vi "Maize traits Extraction_English version.vi"() -> ()   [LabVIEW 2015]
uses:
  <vilib>/vision/Image Controls.llb/IMAQ Image.ctl
  <vilib>/Utility/file.llb/Read Delimited Spreadsheet (string).vi
  <vilib>/Utility/file.llb/Read From Spreadsheet File (string).vi
  <vilib>/Utility/file.llb/Write To Spreadsheet File (string).vi
  <vilib>/vision/NI_Vision_Development_Module.lvlib
  Realse/HistProperty.dll
  GLCM.dll
  <vilib>/Analysis/NI_AALBase.lvlib
  FTKToolkit_CPP_VC8.dll
  Realse/imFillRemove.dll
  TotalContoursConvexHull (5).dll
panel:
  out "Path of segmented images storage":path
  in  "Path of data sotrage":path=path "E:/文章投稿/51. 代明球老师-玉米胁迫实验/RGB程序/TEST"
  out "Barcode":string
  out "Path of input image":path=path "K:/玉米考种机上位机程序/12-255/13SD010-4.png"
  in  "Path of original images":path=path "E:/文章投稿/51. 代明球老师-玉米胁迫实验/RGB程序/TEST/Date.txt"
  out "Date":string
  out "LC上半部分均值":dbl format="%0.2f"
  out "LC上半部分标准差":dbl format="%0.2f"
  out "LC下半部分均值":dbl format="%0.2f"
  out "LC下半部分标准差":dbl format="%0.2f"
  out "叶尖点到结点长度上半部分均值":dbl format="%0.2f"
  out "叶尖点到结点长度上半部分标准差":dbl format="%0.2f"
  out "叶尖点到结点长度下半部分均值":dbl format="%0.2f"
  out "叶尖点到结点长度下半部分标准差":dbl format="%0.2f"
  out "LC均值":dbl format="%0.2f"
  out "LC标准差":dbl format="%0.2f"
  out "叶尖点到结点总长":dbl
  out "叶尖点到结点长度均值":dbl format="%0.2f"
  out "叶尖点到结点长度标准差":dbl format="%0.2f"
  out "steamWidth":dbl
  out "leafEndToEndDistance":dbl[](array[numeric])
  out "unsigned 8bit integer":u8
  out "deleted portion":dbl[](array[numeric])
  out "array w/ subset deleted":dbl[](array[numeric])
  out "拉直后叶长上半部分均值":dbl format="%0.2f"
  out "拉直后叶长上半部分标准差":dbl format="%0.2f"
  out "拉直后叶长下半部分均值":dbl format="%0.2f"
  out "拉直后叶长下半部分标准差":dbl format="%0.2f"
  out "叶片角度2上半部分均值":dbl format="%0.2f"
  out "叶片角度2上半部分标准差":dbl format="%0.2f"
  out "叶片角度2下半部分均值":dbl format="%0.2f"
  out "叶片角度2下半部分标准差":dbl format="%0.2f"
  out "叶片角度1下半部分均值":dbl format="%0.2f"
  out "叶片角度1下半部分标准差":dbl format="%0.2f"
  out "叶片角度1上半部分均值":dbl format="%0.2f"
  out "叶片角度1上半部分标准差":dbl format="%0.2f"
  out "拉直后叶长标准差":dbl format="%0.2f"
  out "拉直后叶长均值":dbl format="%0.2f"
  out "拉直后叶长总长":dbl
  out "叶片角度2总长":dbl format="%0.2f"
  out "叶片角度2标准差":dbl format="%0.2f"
  out "叶片角度1总长(切线)":dbl format="%0.2f"
  out "叶片角度1标准差(切线)":dbl format="%0.2f"
  out "结点长标准差":dbl format="%0.2f"
  out "结点长均值":dbl format="%0.2f"
  out "结点总长":dbl
  out "Convex Hull image":T1(plugin-control)
  out "Gradient image of green component":T1(plugin-control)
  out "leafLength":dbl[](array[numeric])
  out "nodePointPosition":u32[](array[numeric])
  out "leafAngle2":dbl[](array[numeric])
  out "leafAngle1":dbl[](array[numeric])
  out "inputLeafEndPoint":u32[](array[numeric])
  out "outputLeafNum":u32
  out "Area/convex hull area":dbl
  out "Type":dbl
  out "Heywood":dbl
  out "Compactness":dbl
  out "Elongation":dbl
  out "Type_convex hull":dbl
  out "Heywood_convex hull":dbl
  out "Compactness_convex hull":dbl
  out "Elongation_convex hull":dbl
  out "Perimeter_convex hull":dbl
  out "Area_convex hull":dbl
  out "T":sgl[](array[numeric])=[0.2502537, 0.67057997, 5.4486604, 0.09361785, 0.21617743, 888061250.0, 3.9959273, 60957.523, 1.6065311, -402198.06, 2.7884297, 7.334512, 0.26611477, 1.6175103, 60956.69]
  in  "level":i32=16
  out "HistStat_I":dbl[](array[numeric])
  out "HistStat_S":dbl[](array[numeric])
  out "HistStat_G":dbl[](array[numeric])
  out "HistStat_H":dbl[](array[numeric])
  out "GCV2":dbl
  out "HWR":dbl
  out "PP":dbl
  out "FDIC":sgl
  out "TPA":dbl
  out "TBR":dbl
  out "FDNIC":sgl
  out "MPH":dbl
  out "PW":dbl
  out "PAR":dbl
  out "PC1-PC6":sgl[](array[numeric])
  in  "Range":cluster{"Lower value":sgl, "Upper value":sgl}={"Lower value"=110.0, "Upper value"=255.0}
  out "filenames":string[](array[string])
  out "max index(es)":i32
  in  "Removeareathreshold":i32=1000
  in  "EGthreshold":sgl=0.15
  in  "ERthreshold":sgl=0.5
  out "20 side-view images":T1(plugin-control)
  out "Numeric":i32
  out "Original image with maximum plant width":T1(plugin-control)
  out "Segmented image":T1(plugin-control)
  # "Maize Phenotypic traits Extraction"
  # "Plant Traits"
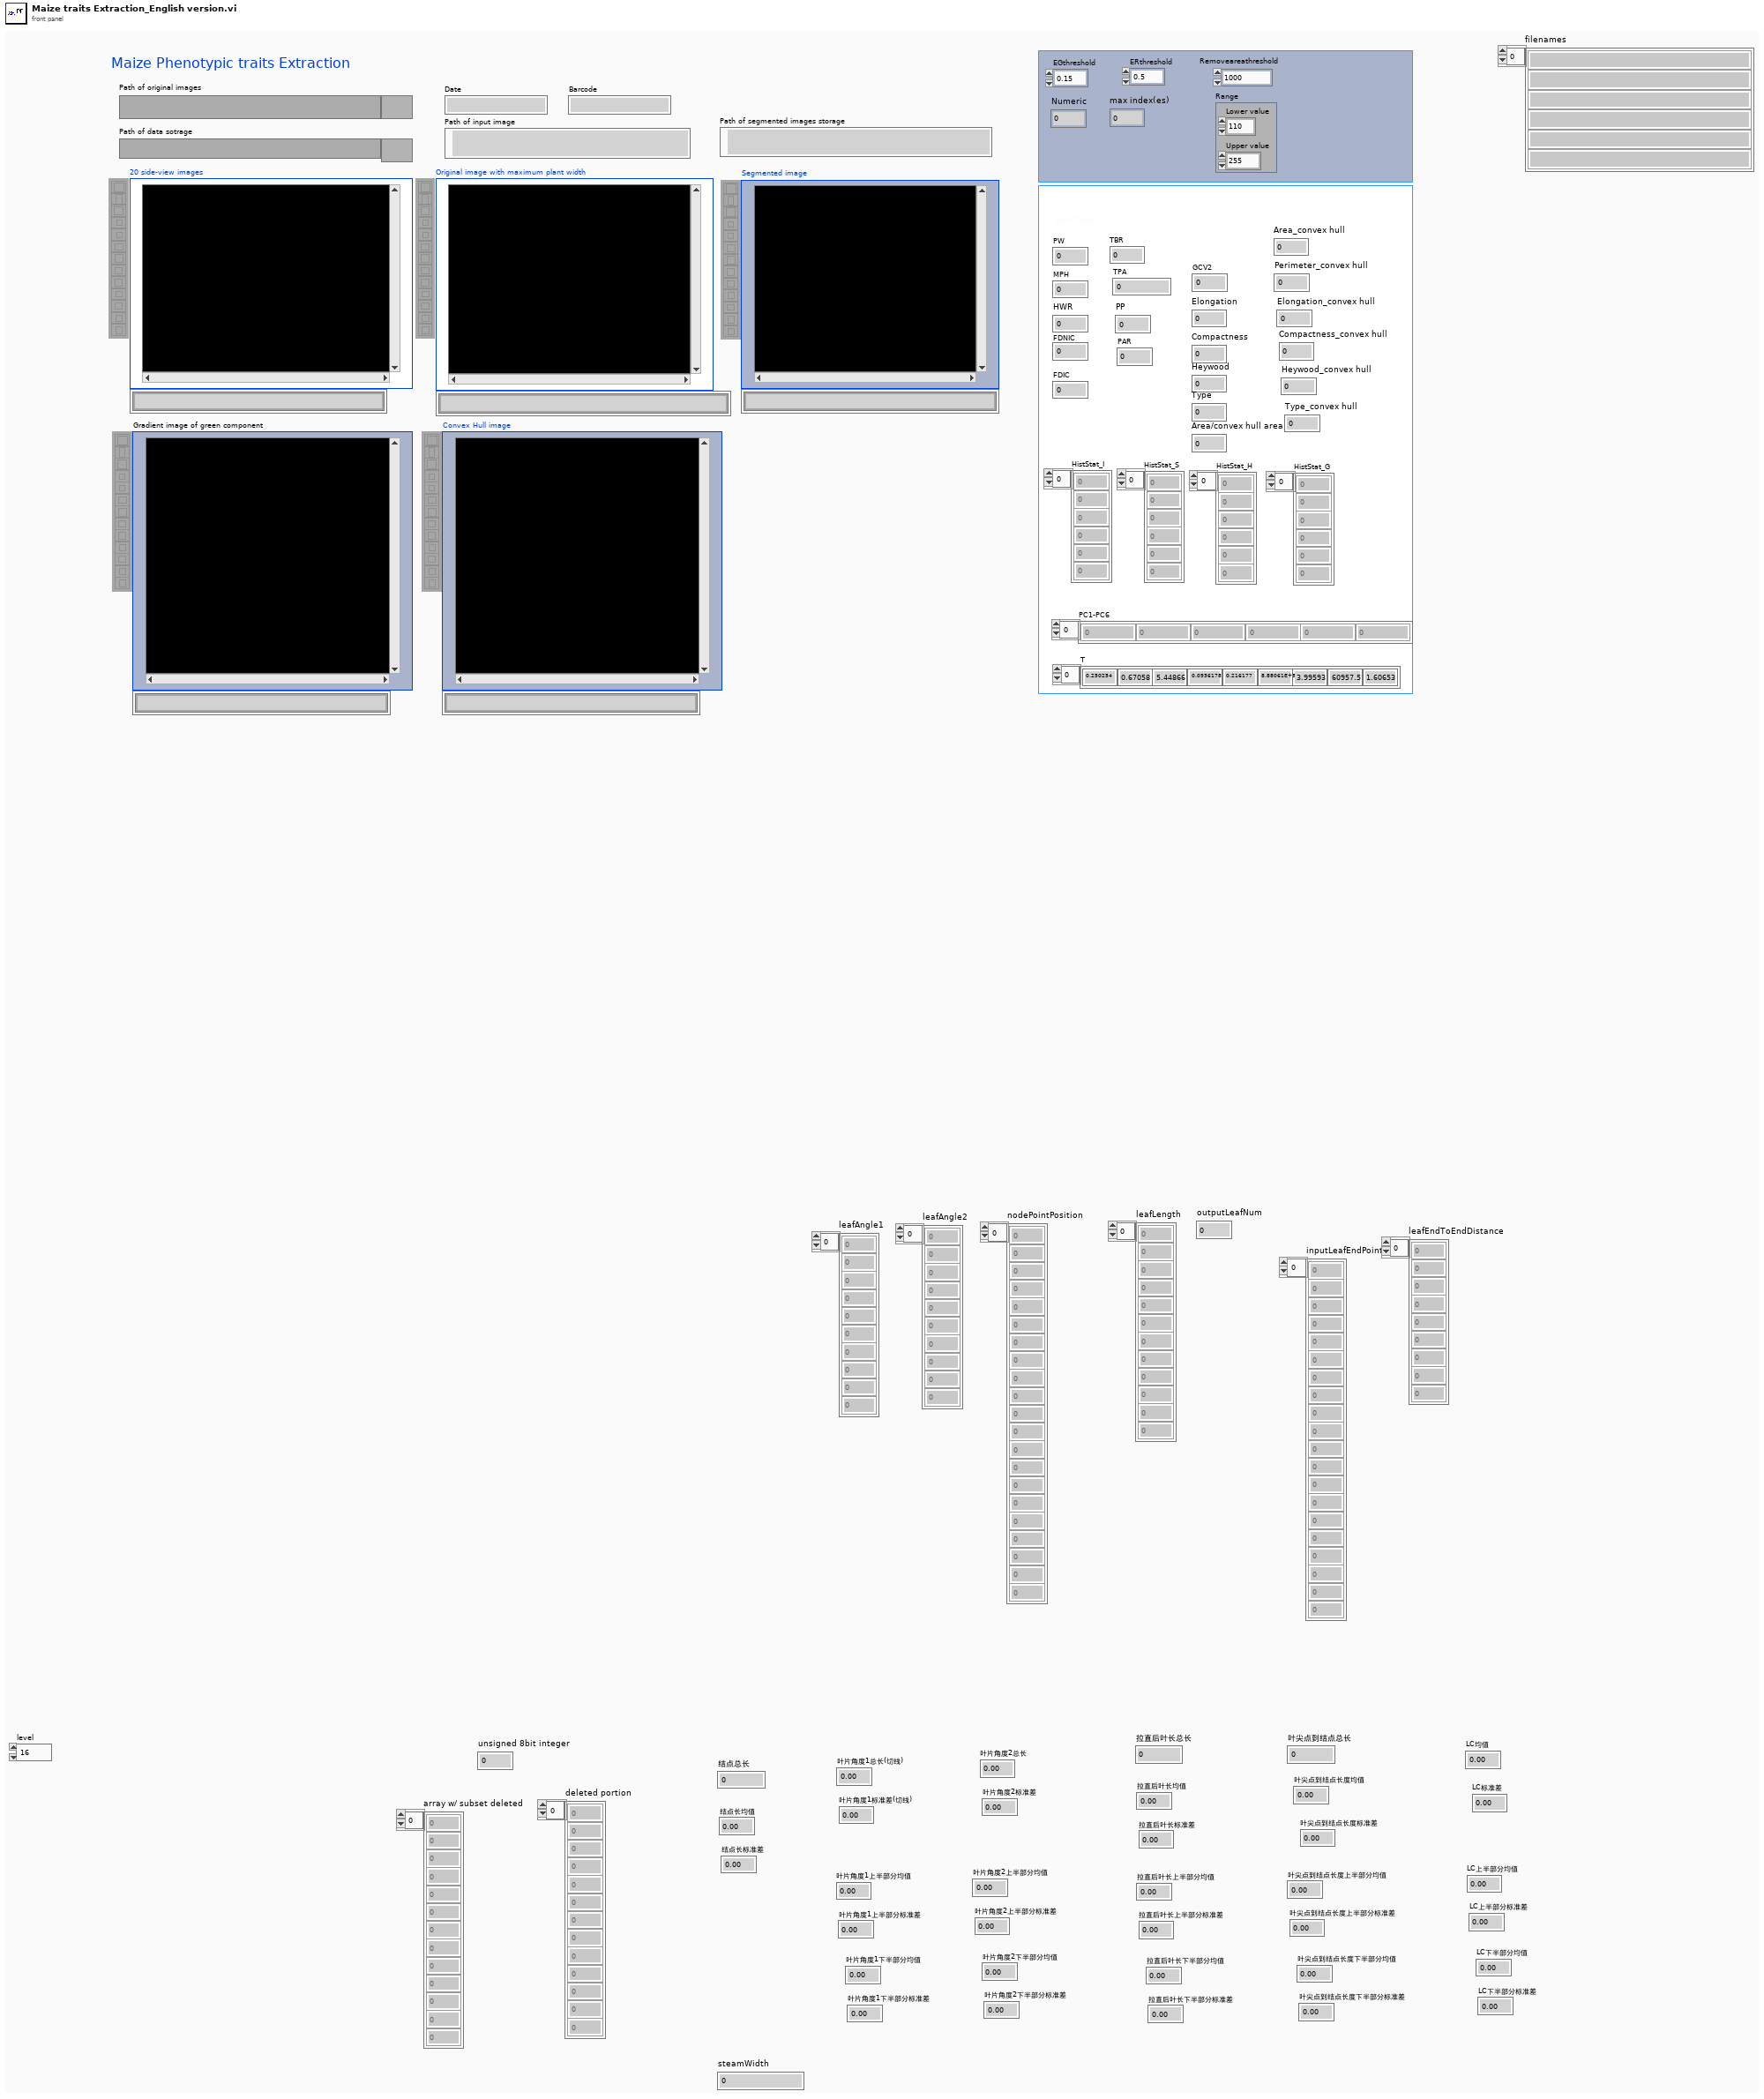
[diagram p1: front panel]
types:
  T1 = typedef "IMAQ Image.ctl" = refnum<image>
  T2 = enum32{"AutoM", "Close", "Dilate", "Erode", "Gradient", "Gradient out", "Gradient in", "Hit miss", "Open", "PClose", "POpen", "Thick", "Thin"}
  T3 = enum32{"AutoM", "Close", "Dilate", "Erode", "Gradient", "Gradient in", "Gradient out", "HitMiss", "Open", "PClose", "POpen", "Thick", "Thin"}
  T4 = typedef "Image Type" = u32
  T5 = typedef "Particle Parameters" = i32
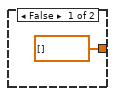
[diagram p2: hidden frame]
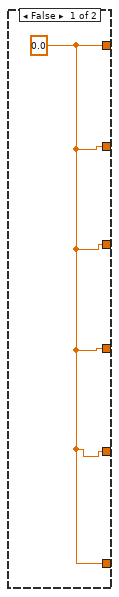
[diagram p3: hidden frame]
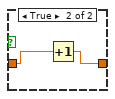
[diagram p7: hidden frame]
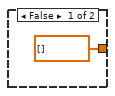
[diagram p8: hidden frame]
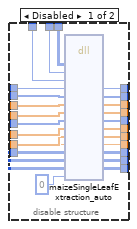
[diagram p10: hidden frame]
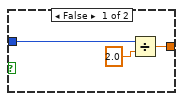
[diagram p11: hidden frame]
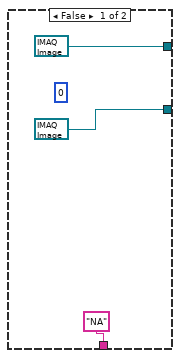
[diagram p13: hidden frame]
diagram:
  n1 = call-poly <vilib>:"Read Delimited Spreadsheet.vi"("file path (dialog if empty)"="Path of original images") -> ("all rows"=w1:string[][])  [unwired: 9 in, 5 out]
  n2 = for {
    tunnel: w1 -> [w14] mode=indexing
    n3 = Index Array(array=w14, index=0) -> (element=w4:string)
    n4 = Reverse String(1:w4) -> (0:w7:string)
    n5 = String To Path(string=w4) -> (path=w8:path)
    n6 = Search/Split String(string=w7, search string/char (-)="\\") -> (substring before match=w5:string)  [unwired: 3 out]
    n7 = Build Path(base path=w8, name or relative path="barcode1.txt") -> (appended path=w17:path)
    n8 = Reverse String(1:w5) -> (0:→"Date":string)
    n9 = Build Path(base path=w8, name or relative path="二值图和骨架图1" ("prompt (Create Folder)")) -> (appended path=w10:path)
    n10 = Create Folder(path (use dialog)=w10) -> (created path=→"Path of segmented images storage":path, error out=w9:errorcluster)  [unwired: 1 in, 2 out]
    n11 = call-poly <vilib>:"Read From Spreadsheet File.vi"("file path (dialog if empty)"=w17) -> ("all rows"=w13:string[][])  [unwired: 3 in, 7 out]
    n12 = Index Array(array=w13, index (col)=0 ("index")) -> (element=w19:string[])  [unwired: 1 in]
    n13 = Array Size(array=w19) -> ()  [unwired: 1 out]
    n14 = call <vilib>:"Clear Errors.vi"("error in (no error)"=w9) -> ()  [unwired: 1 in, 6 out]
    n15 = for {
      tunnel: w13 -> [w29] mode=indexing
      tunnel: w8 -> [w25]
      n16 = Index Array(array=w29, index=0) -> (element=w27:string)
      n17 = flat-sequence {
        tunnel: [w567] -> w36
        tunnel: [w564] -> w37
        tunnel: [w563] -> w28
        tunnel: w27 -> [w563]
        tunnel: [w562] -> w26
        tunnel: w25 -> [w562]
        tunnel: w37 -> [w595]
        tunnel: w36 -> [w596]
        tunnel: [w590] -> w34
        tunnel: [w591] -> w32
        tunnel: [w590] -> w33
        tunnel: [w578] -> w31
        tunnel: w28 -> [w576]
        tunnel: w26 -> [w574]
        tunnel: [w573] -> w24
        tunnel: [w571] -> w21
        tunnel: [w570] -> w20
        frame #0 {
          w566 = T4 4 items=["Grayscale (U8)", "Grayscale (I16)", "Grayscale (SGL)", "Complex (CSG)", "RGB (U32)", "HSL (U32)", "RGB (U64)", "Grayscale (U16)"] ("Image Type")
          w568 = T4 0 items=["Grayscale (U8)", "Grayscale (I16)", "Grayscale (SGL)", "Complex (CSG)", "RGB (U32)", "HSL (U32)", "RGB (U64)", "Grayscale (U16)"] ("Image Type")
          n18 = call "IMAQ Create"("Image Name"="BW", "Image Type"=w568) -> ("New Image"=w567:T1)  [unwired: 2 in, 2 out]
          n19 = call "IMAQ Create"("Image Name"="original", "Image Type"=w566) -> ("New Image"=w564:T1)  [unwired: 2 in, 2 out]
        }
        frame #1 {
          n20 = for {
            N: 20 -> [_]
            tunnel: w596 -> [w674]
            tunnel: [w671] -> w594 mode=indexing
            tunnel: [w670] -> _ mode=indexing
            tunnel: w595 -> [w675]
            tunnel: [w675] -> w593
            tunnel: [w674] -> w592
            tunnel: ["ERthreshold"] -> w582
            tunnel: ["EGthreshold"] -> w581
            tunnel: ["Removeareathreshold"] -> w580
            tunnel: ["Range"] -> w579
            tunnel: w576 -> [w654]
            tunnel: w574 -> [w658]
            tunnel: [w655] -> w575 mode=indexing
            tunnel: [w654] -> w573
            i -> [w657]
            w662 = T4 4 items=["Grayscale (U8)", "Grayscale (I16)", "Grayscale (SGL)", "Complex (CSG)", "RGB (U32)", "HSL (U32)", "RGB (U64)", "Grayscale (U16)"] ("Image Type")
            n21 = call "IMAQ Create"("Image Name"="rgb_original", "Image Type"=w662) -> ("New Image"=w661:T1, "error out"=w660:errorcluster)  [unwired: 2 in, 1 out]
            n22 = Number To Decimal String(number=w657) -> (decimal integer string=w664:string)  [unwired: 1 out]
            n23 = Concatenate Strings(w654, w664, ".png" ("string")) -> (w655:string)
            n24 = Build Path(base path=w658, name or relative path=w655) -> (appended path=w656:path)
            "Path of input image" <- w656
            n25 = call "IMAQ ReadFile"("File Path"=w656, "error in (no error)"=w660, "Image"=w661) -> ("Image Out"=w651:T1)  [unwired: 2 in, 6 out]
            n26 = call "Processing.vi"("Input path"=w656, "BWimag"=w674, "Range"="Range", "ERthreshold"="ERthreshold", "Removeareathreshold"="Removeareathreshold", "EGthreshold"="EGthreshold") -> ("Bwimag"=w673:T1, "original imag"=w672:T1)  [unwired: 4 in, 4 out]
            n27 = call "IMAQ GrayMorphology"("Operation"=T3."Close", "Image Src"=w673) -> ("Image Dst Out"=w669:T1)  [unwired: 5 in, 4 out]
            n28 = call "IMAQ Rotate"("Maintain Size"=FALSE, "Angle (degrees)"=sgl 90.0, "Image Src"=w651) -> ("Image Dst Out"=→"20 side-view images":T1)  [unwired: 5 in, 3 out]
            n29 = call "index.vi"("二值化图像"=w669, "原始图像"=w672) -> ("自然形态宽"=w671:i32, "自然形态高"=w670:i32)  [unwired: 3 out]
            "Numeric" <- w657
            "Barcode" <- w654
          }
          "filenames" <- w575
          n30 = flat-sequence {
            tunnel: [w616] -> w584
            tunnel: w593 -> [w616]
            tunnel: w594 -> [w615]
            tunnel: w592 -> [w610]
            tunnel: [w608] -> w585
            tunnel: [w614] -> w586
            tunnel: [w607] -> w587
            tunnel: [w606] -> w588
            tunnel: [w607] -> w589
            tunnel: w575 -> [w613]
            tunnel: w574 -> [w611]
            tunnel: [w601] -> w583
            tunnel: w582 -> [w605]
            tunnel: w581 -> [w604]
            tunnel: w580 -> [w603]
            tunnel: w579 -> [w602]
            tunnel: [w600] -> w572
            tunnel: [w599] -> w570
            tunnel: w589 -> [w627]
            tunnel: w588 -> [w625]
            tunnel: w587 -> [_]
            tunnel: w586 -> [_]
            tunnel: w585 -> [w628]
            tunnel: w584 -> [w630]
            tunnel: [w621] -> w590
            tunnel: [w620] -> w591
            tunnel: w583 -> [w629]
            tunnel: [w619] -> w578
            tunnel: w572 -> [w618]
            tunnel: [w617] -> w571
            frame #0 {
              # "分割"
              n31 = Array Max & Min(array=w615) -> (max index (indices)=w612:i32, min value=w614:i32)  [unwired: 2 out]
              "max index(es)" <- w612
              n32 = Index Array(array=w613, index=w612) -> (element=w600:string)
              n33 = Build Path(base path=w611, name or relative path=w600) -> (appended path=w609:path)
              n34 = call "Processing.vi"("Input path"=w609, "BWimag"=w610, "Range"=w602, "ERthreshold"=w605, "Removeareathreshold"=w603, "EGthreshold"=w604) -> ("GPAR"=w599:dbl, "Bwimag"=w601:T1, "original imag"=w608:T1)  [unwired: 4 in, 3 out]
              "Original image with maximum plant width" <- w608
              n35 = call "index.vi"("二值化图像"=w601, "原始图像"=w608) -> ("自然形态宽"=w607:i32, "自然形态高"=w606:i32)  [unwired: 3 out]
            }
            frame #1 {
              # "不是空图"
              n36 = Greater?(x=w627, y=100) -> (0:w623:bool)
              n37 = Greater?(x=w625, y=100) -> (0:w622:bool)
              n38 = And(x=w623, y=w622) -> (x .and. y?=w619:bool)
              n39 = case shown="True" w619 {
                tunnel: w630 -> [_ w649]
                tunnel: w629 -> [_ w635]
                tunnel: w628 -> [_ w648]
                tunnel: [T1 refnum ("Image Dst Out") w635] -> w621
                tunnel: [T1 refnum ("Image Dst Out") w647] -> w620
                tunnel: w618 -> [_ w641]
                tunnel: ["NA" w641] -> w617
                frame False {
                  (unwired) 0 ("颜色（2g-r-b）")
                }
                frame True {
                  w638 = T4 0 items=["Grayscale (U8)", "Grayscale (I16)", "Grayscale (SGL)", "Complex (CSG)", "RGB (U32)", "HSL (U32)", "RGB (U64)", "Grayscale (U16)"] ("Image Type")
                  w645 = T4 4 items=["Grayscale (U8)", "Grayscale (I16)", "Grayscale (SGL)", "Complex (CSG)", "RGB (U32)", "HSL (U32)", "RGB (U64)", "Grayscale (U16)"] ("Image Type")
                  n40 = local read "Path of segmented images storage"() -> (w643:path)
                  n41 = call "IMAQ Copy"("Image Dst"=w649, "Image Src"=w648) -> ("Image Dst Out"=w647:T1)  [unwired: 1 in, 4 out]
                  n42 = call "IMAQ Create"("Image Name"="BW_color", "Image Type"=w638) -> ("New Image"=w636:T1)  [unwired: 2 in, 2 out]
                  n43 = call "IMAQ Create"("Image Name"="BW_final", "Image Type"=w645) -> ("New Image"=w644:T1)  [unwired: 2 in, 2 out]
                  n44 = Build Path(base path=w643, name or relative path=w641) -> (appended path=w642:path)
                  n45 = call "IMAQ Copy"("Image Dst"=w644, "Image Src"=w635) -> ("Image Dst Out"=w640:T1)  [unwired: 1 in, 4 out]
                  n46 = call "IMAQ Multiply"("Image Src A"=w640, "Constant"=sgl 255.0, "Image Dst"=w636) -> ("Image Dst Out"=w634:T1)  [unwired: 2 in, 3 out]
                  "Segmented image" <- w634
                  n47 = call-poly "IMAQ Write File 2"("File Path"=w642, "Image"=w634) -> ()  [unwired: 4 in, 6 out]
                }
              }
            }
          }
          n48 = disable-structure shown="Disabled" {
            frame Disabled {
              n49 = call "RegionGrow.vi"() -> ()  [unwired: 2 in, 4 out]
              n50 = call "IMAQ Morphology"("Operation"=T2."Close") -> ("Image Src"=w598:T1)  [unwired: 5 in, 5 out]
            }
            frame Enabled {
            }
          }
        }
      }
      n51 = flat-sequence {
        tunnel: w34 -> [w43]
        tunnel: w33 -> [w41]
        tunnel: w32 -> [w42]
        tunnel: [w43] -> w35
        tunnel: w31 -> [w39]
        tunnel: [w40] -> w23
        tunnel: [w39] -> w22
        tunnel: w20 -> [w38]
        tunnel: w35 -> [w337]
        tunnel: w24 -> [w329]
        tunnel: w23 -> [w327]
        tunnel: w22 -> [w325]
        tunnel: w21 -> [w324]
        frame #0 {
          n52 = case shown="True" w39 {
            tunnel: w43 -> [_ w212]
            tunnel: w42 -> [_ w102]
            tunnel: w41 -> [_ w77]
            tunnel: [dbl[] [] w46] -> w40
            tunnel: w38 -> [_ w45]
            frame False {
            }
            frame True {
              w85 = T5[] [56] items=["Center of Mass X", "Center of Mass Y", "First Pixel X", "First Pixel Y", "Bounding Rect Left", "Bounding Rect Top", "Bounding Rect Right", "Bounding Rect Bottom", "Max Feret Diameter Start X", "Max Feret Diameter Start Y", "Max Feret Diameter End X", "Max Feret Diameter End Y", "Max Horiz. Segment Length Left", "Max Horiz. Segment Length Right", "Max Horiz. Segment Length Row", "-", "Bounding Rect Width", "Bounding Rect Height", "Bounding Rect Diagonal", "Perimeter", "Convex Hull Perimeter", "Holes' Perimeter", "Max Feret Diameter", "Equivalent Ellipse Major Axis", "Equivalent Ellipse Minor Axis", "Equivalent Ellipse Minor Axis (Feret)", "Equivalent Rect Long Side", "Equivalent Rect Short Side", "Equivalent Rect Diagonal", "Equivalent Rect Short Side (Feret)", "Average Horiz. Segment Length", "Average Vert. Segment Length", "Hydraulic Radius", "Waddel Disk Diameter", "-", "Area", "Holes' Area", "Particle & Holes' Area", "Convex Hull Area", "Image Area", "-", "Number of Holes", "Number of Horiz. Segments", "Number of Vert. Segments", "-", "Orientation", "Max Feret Diameter Orientation", "-", "% Area/Image Area", "% Area/(Particle & Holes' Area)", "Ratio of Equivalent Ellipse Axes", "Ratio of Equivalent Rect Sides", "-", "Elongation Factor", "Compactness Factor", "Heywood Circularity Factor", "Type Factor", "-", "Sum X", "Sum Y", "Sum XX", "Sum XY", "Sum YY", "Sum XXX", "Sum XXY", "Sum XYY", "Sum YYY", "-", "Moment of Inertia XX", "Moment of Inertia XY", "Moment of Inertia YY", "Moment of Inertia XXX", "Moment of Inertia XXY", "Moment of Inertia XYY", "Moment of Inertia YYY", "Norm. Moment of Inertia XX", "Norm. Moment of Inertia XY", "Norm. Moment of Inertia YY", "Norm. Moment of Inertia XXX", "Norm. Moment of Inertia XXY", "Norm. Moment of Inertia XYY", "Norm. Moment of Inertia YYY", "Hu Moment 1", "Hu Moment 2", "Hu Moment 3", "Hu Moment 4", "Hu Moment 5", "Hu Moment 6", "Hu Moment 7"] ("Pixel Measurements")
              w89 = T5[] [55] items=["Center of Mass X", "Center of Mass Y", "First Pixel X", "First Pixel Y", "Bounding Rect Left", "Bounding Rect Top", "Bounding Rect Right", "Bounding Rect Bottom", "Max Feret Diameter Start X", "Max Feret Diameter Start Y", "Max Feret Diameter End X", "Max Feret Diameter End Y", "Max Horiz. Segment Length Left", "Max Horiz. Segment Length Right", "Max Horiz. Segment Length Row", "-", "Bounding Rect Width", "Bounding Rect Height", "Bounding Rect Diagonal", "Perimeter", "Convex Hull Perimeter", "Holes' Perimeter", "Max Feret Diameter", "Equivalent Ellipse Major Axis", "Equivalent Ellipse Minor Axis", "Equivalent Ellipse Minor Axis (Feret)", "Equivalent Rect Long Side", "Equivalent Rect Short Side", "Equivalent Rect Diagonal", "Equivalent Rect Short Side (Feret)", "Average Horiz. Segment Length", "Average Vert. Segment Length", "Hydraulic Radius", "Waddel Disk Diameter", "-", "Area", "Holes' Area", "Particle & Holes' Area", "Convex Hull Area", "Image Area", "-", "Number of Holes", "Number of Horiz. Segments", "Number of Vert. Segments", "-", "Orientation", "Max Feret Diameter Orientation", "-", "% Area/Image Area", "% Area/(Particle & Holes' Area)", "Ratio of Equivalent Ellipse Axes", "Ratio of Equivalent Rect Sides", "-", "Elongation Factor", "Compactness Factor", "Heywood Circularity Factor", "Type Factor", "-", "Sum X", "Sum Y", "Sum XX", "Sum XY", "Sum YY", "Sum XXX", "Sum XXY", "Sum XYY", "Sum YYY", "-", "Moment of Inertia XX", "Moment of Inertia XY", "Moment of Inertia YY", "Moment of Inertia XXX", "Moment of Inertia XXY", "Moment of Inertia XYY", "Moment of Inertia YYY", "Norm. Moment of Inertia XX", "Norm. Moment of Inertia XY", "Norm. Moment of Inertia YY", "Norm. Moment of Inertia XXX", "Norm. Moment of Inertia XXY", "Norm. Moment of Inertia XYY", "Norm. Moment of Inertia YYY", "Hu Moment 1", "Hu Moment 2", "Hu Moment 3", "Hu Moment 4", "Hu Moment 5", "Hu Moment 6", "Hu Moment 7"] ("Pixel Measurements")
              w87 = T5[] [54] items=["Center of Mass X", "Center of Mass Y", "First Pixel X", "First Pixel Y", "Bounding Rect Left", "Bounding Rect Top", "Bounding Rect Right", "Bounding Rect Bottom", "Max Feret Diameter Start X", "Max Feret Diameter Start Y", "Max Feret Diameter End X", "Max Feret Diameter End Y", "Max Horiz. Segment Length Left", "Max Horiz. Segment Length Right", "Max Horiz. Segment Length Row", "-", "Bounding Rect Width", "Bounding Rect Height", "Bounding Rect Diagonal", "Perimeter", "Convex Hull Perimeter", "Holes' Perimeter", "Max Feret Diameter", "Equivalent Ellipse Major Axis", "Equivalent Ellipse Minor Axis", "Equivalent Ellipse Minor Axis (Feret)", "Equivalent Rect Long Side", "Equivalent Rect Short Side", "Equivalent Rect Diagonal", "Equivalent Rect Short Side (Feret)", "Average Horiz. Segment Length", "Average Vert. Segment Length", "Hydraulic Radius", "Waddel Disk Diameter", "-", "Area", "Holes' Area", "Particle & Holes' Area", "Convex Hull Area", "Image Area", "-", "Number of Holes", "Number of Horiz. Segments", "Number of Vert. Segments", "-", "Orientation", "Max Feret Diameter Orientation", "-", "% Area/Image Area", "% Area/(Particle & Holes' Area)", "Ratio of Equivalent Ellipse Axes", "Ratio of Equivalent Rect Sides", "-", "Elongation Factor", "Compactness Factor", "Heywood Circularity Factor", "Type Factor", "-", "Sum X", "Sum Y", "Sum XX", "Sum XY", "Sum YY", "Sum XXX", "Sum XXY", "Sum XYY", "Sum YYY", "-", "Moment of Inertia XX", "Moment of Inertia XY", "Moment of Inertia YY", "Moment of Inertia XXX", "Moment of Inertia XXY", "Moment of Inertia XYY", "Moment of Inertia YYY", "Norm. Moment of Inertia XX", "Norm. Moment of Inertia XY", "Norm. Moment of Inertia YY", "Norm. Moment of Inertia XXX", "Norm. Moment of Inertia XXY", "Norm. Moment of Inertia XYY", "Norm. Moment of Inertia YYY", "Hu Moment 1", "Hu Moment 2", "Hu Moment 3", "Hu Moment 4", "Hu Moment 5", "Hu Moment 6", "Hu Moment 7"] ("Pixel Measurements")
              w92 = T5[] [53] items=["Center of Mass X", "Center of Mass Y", "First Pixel X", "First Pixel Y", "Bounding Rect Left", "Bounding Rect Top", "Bounding Rect Right", "Bounding Rect Bottom", "Max Feret Diameter Start X", "Max Feret Diameter Start Y", "Max Feret Diameter End X", "Max Feret Diameter End Y", "Max Horiz. Segment Length Left", "Max Horiz. Segment Length Right", "Max Horiz. Segment Length Row", "-", "Bounding Rect Width", "Bounding Rect Height", "Bounding Rect Diagonal", "Perimeter", "Convex Hull Perimeter", "Holes' Perimeter", "Max Feret Diameter", "Equivalent Ellipse Major Axis", "Equivalent Ellipse Minor Axis", "Equivalent Ellipse Minor Axis (Feret)", "Equivalent Rect Long Side", "Equivalent Rect Short Side", "Equivalent Rect Diagonal", "Equivalent Rect Short Side (Feret)", "Average Horiz. Segment Length", "Average Vert. Segment Length", "Hydraulic Radius", "Waddel Disk Diameter", "-", "Area", "Holes' Area", "Particle & Holes' Area", "Convex Hull Area", "Image Area", "-", "Number of Holes", "Number of Horiz. Segments", "Number of Vert. Segments", "-", "Orientation", "Max Feret Diameter Orientation", "-", "% Area/Image Area", "% Area/(Particle & Holes' Area)", "Ratio of Equivalent Ellipse Axes", "Ratio of Equivalent Rect Sides", "-", "Elongation Factor", "Compactness Factor", "Heywood Circularity Factor", "Type Factor", "-", "Sum X", "Sum Y", "Sum XX", "Sum XY", "Sum YY", "Sum XXX", "Sum XXY", "Sum XYY", "Sum YYY", "-", "Moment of Inertia XX", "Moment of Inertia XY", "Moment of Inertia YY", "Moment of Inertia XXX", "Moment of Inertia XXY", "Moment of Inertia XYY", "Moment of Inertia YYY", "Norm. Moment of Inertia XX", "Norm. Moment of Inertia XY", "Norm. Moment of Inertia YY", "Norm. Moment of Inertia XXX", "Norm. Moment of Inertia XXY", "Norm. Moment of Inertia XYY", "Norm. Moment of Inertia YYY", "Hu Moment 1", "Hu Moment 2", "Hu Moment 3", "Hu Moment 4", "Hu Moment 5", "Hu Moment 6", "Hu Moment 7"] ("Pixel Measurements")
              w101 = T5[] [35] items=["Center of Mass X", "Center of Mass Y", "First Pixel X", "First Pixel Y", "Bounding Rect Left", "Bounding Rect Top", "Bounding Rect Right", "Bounding Rect Bottom", "Max Feret Diameter Start X", "Max Feret Diameter Start Y", "Max Feret Diameter End X", "Max Feret Diameter End Y", "Max Horiz. Segment Length Left", "Max Horiz. Segment Length Right", "Max Horiz. Segment Length Row", "-", "Bounding Rect Width", "Bounding Rect Height", "Bounding Rect Diagonal", "Perimeter", "Convex Hull Perimeter", "Holes' Perimeter", "Max Feret Diameter", "Equivalent Ellipse Major Axis", "Equivalent Ellipse Minor Axis", "Equivalent Ellipse Minor Axis (Feret)", "Equivalent Rect Long Side", "Equivalent Rect Short Side", "Equivalent Rect Diagonal", "Equivalent Rect Short Side (Feret)", "Average Horiz. Segment Length", "Average Vert. Segment Length", "Hydraulic Radius", "Waddel Disk Diameter", "-", "Area", "Holes' Area", "Particle & Holes' Area", "Convex Hull Area", "Image Area", "-", "Number of Holes", "Number of Horiz. Segments", "Number of Vert. Segments", "-", "Orientation", "Max Feret Diameter Orientation", "-", "% Area/Image Area", "% Area/(Particle & Holes' Area)", "Ratio of Equivalent Ellipse Axes", "Ratio of Equivalent Rect Sides", "-", "Elongation Factor", "Compactness Factor", "Heywood Circularity Factor", "Type Factor", "-", "Sum X", "Sum Y", "Sum XX", "Sum XY", "Sum YY", "Sum XXX", "Sum XXY", "Sum XYY", "Sum YYY", "-", "Moment of Inertia XX", "Moment of Inertia XY", "Moment of Inertia YY", "Moment of Inertia XXX", "Moment of Inertia XXY", "Moment of Inertia XYY", "Moment of Inertia YYY", "Norm. Moment of Inertia XX", "Norm. Moment of Inertia XY", "Norm. Moment of Inertia YY", "Norm. Moment of Inertia XXX", "Norm. Moment of Inertia XXY", "Norm. Moment of Inertia XYY", "Norm. Moment of Inertia YYY", "Hu Moment 1", "Hu Moment 2", "Hu Moment 3", "Hu Moment 4", "Hu Moment 5", "Hu Moment 6", "Hu Moment 7"] ("Pixel Measurements")
              w105 = T4 0 items=["Grayscale (U8)", "Grayscale (I16)", "Grayscale (SGL)", "Complex (CSG)", "RGB (U32)", "HSL (U32)", "RGB (U64)", "Grayscale (U16)"] ("Image Type")
              w112 = T4 0 items=["Grayscale (U8)", "Grayscale (I16)", "Grayscale (SGL)", "Complex (CSG)", "RGB (U32)", "HSL (U32)", "RGB (U64)", "Grayscale (U16)"] ("Image Type")
              w114 = T4 0 items=["Grayscale (U8)", "Grayscale (I16)", "Grayscale (SGL)", "Complex (CSG)", "RGB (U32)", "HSL (U32)", "RGB (U64)", "Grayscale (U16)"] ("Image Type")
              w116 = 1 items=["Red", "Green", "Blue", "Hue", "Saturation", "Luminance", "Value", "Intensity"] ("Color Plane")
              w155 = T4 0 items=["Grayscale (U8)", "Grayscale (I16)", "Grayscale (SGL)", "Complex (CSG)", "RGB (U32)", "HSL (U32)", "RGB (U64)", "Grayscale (U16)"] ("Image Type")
              w160 = T4 0 items=["Grayscale (U8)", "Grayscale (I16)", "Grayscale (SGL)", "Complex (CSG)", "RGB (U32)", "HSL (U32)", "RGB (U64)", "Grayscale (U16)"] ("Image Type")
              w161 = 4 items=["Red", "Green", "Blue", "Hue", "Saturation", "Luminance", "Value", "Intensity"] ("Color Plane")
              w174 = T4 0 items=["Grayscale (U8)", "Grayscale (I16)", "Grayscale (SGL)", "Complex (CSG)", "RGB (U32)", "HSL (U32)", "RGB (U64)", "Grayscale (U16)"] ("Image Type")
              w179 = T4 0 items=["Grayscale (U8)", "Grayscale (I16)", "Grayscale (SGL)", "Complex (CSG)", "RGB (U32)", "HSL (U32)", "RGB (U64)", "Grayscale (U16)"] ("Image Type")
              w180 = 1 items=["Red", "Green", "Blue", "Hue", "Saturation", "Luminance", "Value", "Intensity"] ("Color Plane")
              w193 = T4 0 items=["Grayscale (U8)", "Grayscale (I16)", "Grayscale (SGL)", "Complex (CSG)", "RGB (U32)", "HSL (U32)", "RGB (U64)", "Grayscale (U16)"] ("Image Type")
              w198 = T4 0 items=["Grayscale (U8)", "Grayscale (I16)", "Grayscale (SGL)", "Complex (CSG)", "RGB (U32)", "HSL (U32)", "RGB (U64)", "Grayscale (U16)"] ("Image Type")
              w199 = 3 items=["Red", "Green", "Blue", "Hue", "Saturation", "Luminance", "Value", "Intensity"] ("Color Plane")
              w209 = T4 0 items=["Grayscale (U8)", "Grayscale (I16)", "Grayscale (SGL)", "Complex (CSG)", "RGB (U32)", "HSL (U32)", "RGB (U64)", "Grayscale (U16)"] ("Image Type")
              w211 = 1 items=["Red", "Green", "Blue", "Hue", "Saturation", "Luminance", "Value", "Intensity"] ("Color Plane")
              w216 = 7 items=["Red", "Green", "Blue", "Hue", "Saturation", "Luminance", "Value", "Intensity"] ("Color Plane")
              w214 = T4 0 items=["Grayscale (U8)", "Grayscale (I16)", "Grayscale (SGL)", "Complex (CSG)", "RGB (U32)", "HSL (U32)", "RGB (U64)", "Grayscale (U16)"] ("Image Type")
              # "凸包6个性状"
              # "计算纹理特征"
              # "计算性状"
              n53 = call "IMAQ Create"("Image Name"="gard2", "Image Type"=w112) -> ("New Image"=w110:T1)  [unwired: 2 in, 2 out]
              n54 = call "IMAQ Create"("Image Name"="gard1", "Image Type"=w114) -> ("New Image"=w113:T1)  [unwired: 2 in, 2 out]
              n55 = call "IMAQ ImageToArray"("Image"=w77) -> ("Image Pixels (U8)"=w107:u8[][])  [unwired: 2 in, 5 out]
              n56 = call "IMAQ Create"("Image Name"="Intensity_H", "Image Type"=w198) -> ("New Image"=w196:T1)  [unwired: 2 in, 2 out]
              n57 = call "IMAQ Create"("Image Name"="Intensity_G", "Image Type"=w179) -> ("New Image"=w177:T1)  [unwired: 2 in, 2 out]
              n58 = call "IMAQ Create"("Image Name"="Intensity_S", "Image Type"=w160) -> ("New Image"=w158:T1)  [unwired: 2 in, 2 out]
              n59 = call "IMAQ GetImageSize"("Image"=w102) -> ("Y Resolution"=w109:i32, "X Resolution"=w108:i32)  [unwired: 1 in, 3 out]
              n60 = Initialize Array(sgl 0.0 ("element"), 1816 ("dimension size"), 1730 ("dimension size 2")) -> (w232:sgl[][])
              n61 = call "IMAQ ExtractSingleColorPlane"("Color Plane"=w199, "Image Dst"=w196, "Image Src"=w102) -> ("Image Dst Out"=w195:T1)  [unwired: 1 in, 7 out]
              n62 = call "IMAQ ExtractSingleColorPlane"("Color Plane"=w180, "Image Dst"=w177, "Image Src"=w102) -> ("Image Dst Out"=w176:T1)  [unwired: 1 in, 7 out]
              n63 = call "IMAQ ExtractSingleColorPlane"("Color Plane"=w161, "Image Dst"=w158, "Image Src"=w102) -> ("Image Dst Out"=w157:T1)  [unwired: 1 in, 7 out]
              n64 = call "IMAQ Create"("Image Name"="G2", "Image Type"=w209) -> ("New Image"=w208:T1)  [unwired: 2 in, 2 out]
              n65 = call "DensityCalculation.vi"("dens"=w232, "bw image"=w212) -> ("dens output"=w231:sgl[][])  [unwired: 2 out]
              n66 = call "FeaturesCalculation.vi"("bw"=w212) -> ("PP"=w67:dbl, "FDIC"=w68:sgl, "PAR"=w74:dbl, "PW"=w73:dbl, "MPH"=w72:dbl, "TPA"=w69:dbl, "FDNIC"=w71:sgl, "TBR"=w70:dbl)  [unwired: 2 out]
              "PAR" <- w74
              "PW" <- w73
              "MPH" <- w72
              "FDNIC" <- w71
              "TBR" <- w70
              "TPA" <- w69
              "FDIC" <- w68
              "PP" <- w67
              n67 = call "RatioCalculation.vi"("dens"=w231) -> ("ratio"=w75:sgl[])  [unwired: 2 out]
              "PC1-PC6" <- w75
              n68 = call "IMAQ ExtractSingleColorPlane"("Color Plane"=w211, "Image Dst"=w208, "Image Src"=w102) -> ("Image Dst Out"=w200:T1)  [unwired: 1 in, 7 out]
              n69 = call "IMAQ ExtractSingleColorPlane"("Color Plane"=w116, "Image Dst"=w113, "Image Src"=w102) -> ("Image Dst Out"=w139:T1)  [unwired: 1 in, 7 out]
              n70 = call "IMAQ Create"("Image Name"="Intensity1_H", "Image Type"=w193) -> ("New Image"=w192:T1)  [unwired: 2 in, 2 out]
              n71 = call "IMAQ Create"("Image Name"="Intensity1_G", "Image Type"=w174) -> ("New Image"=w173:T1)  [unwired: 2 in, 2 out]
              n72 = call "IMAQ ImageToArray"("Image"=w200) -> ("Image Pixels (U8)"=w207:u8[][])  [unwired: 2 in, 5 out]
              n73 = call "IMAQ Create"("Image Name"="Intensity1_S", "Image Type"=w155) -> ("New Image"=w154:T1)  [unwired: 2 in, 2 out]
              n74 = call "IMAQ ImageToArray"("Image"=w139) -> ("Image Pixels (U8)"=w135:u8[][])  [unwired: 2 in, 5 out]
              n75 = call "IMAQ Convolute"("Kernel"=sgl[][] [[-1.0, -1.0, -1.0], [-1.0, 8.0, -1.0], [-1.0, -1.0, -1.0]], "Image Dst"=w110, "Image Src"=w139) -> ("Image Dst Out"=w142:T1)  [unwired: 4 in, 4 out]
              n76 = Divide(x=w72, y=w73) -> (x/y=w66:dbl)
              "HWR" <- w66
              n77 = Array Max & Min(array=w135) -> (max value=w127:u8)  [unwired: 3 out]
              n78 = call "IMAQ ImageToArray"("Image"=w142) -> ("Image Pixels (U8)"=w140:u8[][])  [unwired: 2 in, 5 out]
              n79 = call "IMAQ Multiply"("Image Src A"=w77, "Image Dst"=w192, "Image Src B"=w195) -> ("Image Dst Out"=w181:T1)  [unwired: 2 in, 3 out]
              n80 = call "IMAQ Create"("Image Name"="Intensity_I", "Image Type"=w214) -> ("New Image"=w215:T1)  [unwired: 2 in, 2 out]
              n81 = call "IMAQ Multiply"("Image Src A"=w77, "Image Dst"=w173, "Image Src B"=w176) -> ("Image Dst Out"=w162:T1)  [unwired: 2 in, 3 out]
              n82 = call "IMAQ GetImageSize"("Image"=w200) -> ("Y Resolution"=w204:i32, "X Resolution"=w205:i32)  [unwired: 1 in, 3 out]
              n83 = call "IMAQ Multiply"("Image Src A"=w77, "Image Dst"=w154, "Image Src B"=w157) -> ("Image Dst Out"=w144:T1)  [unwired: 2 in, 3 out]
              n84 = call "IMAQ ExtractSingleColorPlane"("Color Plane"=w216, "Image Dst"=w215, "Image Src"=w102) -> ("Image Dst Out"=w228:T1)  [unwired: 1 in, 7 out]
              n85 = Multiply(x=w140, y=w107) -> (x*y=w103:u8[][])
              n86 = Decrement(x="level") -> (x-1=w126:i32)
              n87 = call "IMAQ Create"("Image Name"="gard3", "Image Type"=w105) -> ("New Image"=w104:T1)  [unwired: 2 in, 2 out]
              n88 = call "IMAQ Multiply"("Image Src A"=w228, "Image Dst"=w228, "Image Src B"=w77) -> ("Image Dst Out"=w229:T1)  [unwired: 2 in, 3 out]
              n89 = Multiply(x=w126, y=w135) -> (x*y=w134:i32[][])
              n90 = Array Max & Min(array=w103) -> (max value=w118:u8)  [unwired: 3 out]
              n91 = call "IMAQ ImageToArray"("Image"=w229) -> ("error out"=w225:errorcluster, "Image Pixels (U8)"=w217:u8[][])  [unwired: 2 in, 4 out]
              n92 = call "IMAQ GetImageSize"("Image"=w229) -> ("Y Resolution"=w230:i32, "X Resolution"=w220:i32)  [unwired: 1 in, 3 out]
              n93 = call "IMAQ ImageToArray"("Image"=w181) -> ("error out"=w182:errorcluster, "Image Pixels (U8)"=w191:u8[][])  [unwired: 2 in, 4 out]
              n94 = call "IMAQ ImageToArray"("Image"=w162) -> ("error out"=w163:errorcluster, "Image Pixels (U8)"=w172:u8[][])  [unwired: 2 in, 4 out]
              n95 = call "IMAQ ImageToArray"("Image"=w144) -> ("error out"=w145:errorcluster, "Image Pixels (U8)"=w143:u8[][])  [unwired: 2 in, 4 out]
              n96 = Multiply(x=w103, y=w126) -> (x*y=w131:i32[][])
              n97 = for {
                N: w205 -> [_]
                tunnel: w207 -> [w311]
                shift-right: [w309] -> w203
                shift-left: u64 0 -> [w306]
                tunnel: w204 -> [w307]
                shift-right: [w303] -> w201
                shift-left: 0.0 -> [w302]
                i -> [w308]
                n98 = for {
                  N: w307 -> [_]
                  tunnel: w311 -> [w319]
                  shift-right: [w316] -> w310
                  shift-left: u64 0 -> [w320]
                  tunnel: w308 -> [w317]
                  shift-right: [w313] -> w304
                  shift-left: 0.0 -> [w312]
                  i -> [w318]
                  n99 = Index Array(array=w319, index (row)=w318, index (col)=w317) -> (element=w315:u8)
                  n100 = Not Equal To 0?(x=w315) -> (x != 0?=w314:bool)
                  n101 = Add(x=w315, y=w320) -> (x+y=w316:u64)
                  n102 = case shown="False" w314 {
                    tunnel: [w321 w323] -> w313
                    tunnel: w312 -> [w321 w322]
                    frame False {
                    }
                    frame True {
                      n103 = Increment(x=w322) -> (x+1=w323:dbl)
                    }
                  }
                }
                n104 = Add(x=w304, y=w302) -> (x+y=w303:dbl)
                n105 = Add(x=w310, y=w306) -> (x+y=w309:u64)
              }
              n106 = call "IMAQ ArrayToImage"("Image Pixels (U8)"=w103, "Image"=w104) -> ("Image Out"=→"Gradient image of green component":T1)  [unwired: 4 in, 5 out]
              n107 = Divide(x=w134, y=w127) -> (x/y=w124:dbl[][])
              n108 = disable-structure shown="Enabled" {
                disable-tunnel: w191 -> [w299 w300]
                disable-tunnel: u8 8 ("y") -> [w298 _]
                disable-tunnel: [w295 w300] -> w189
                frame Enabled {
                  n109 = Divide(x=w299, y=w298) -> (x/y=w297:dbl[][])
                  n110 = Round Toward -Infinity(1:w297) -> (0:w296:dbl[][])
                  n111 = To Unsigned Byte Integer(number=w296) -> (unsigned 8bit integer=w295:u8[][])
                }
                frame Disabled {
                }
              }
              n112 = Divide(x=w217, y=u8 8) -> (x/y=w226:dbl[][])
              n113 = disable-structure shown="Enabled" {
                disable-tunnel: w172 -> [w293 w294]
                disable-tunnel: u8 8 ("y") -> [w292 _]
                disable-tunnel: [w289 w294] -> w170
                frame Enabled {
                  n114 = Divide(x=w293, y=w292) -> (x/y=w291:dbl[][])
                  n115 = Round Toward -Infinity(1:w291) -> (0:w290:dbl[][])
                  n116 = To Unsigned Byte Integer(number=w290) -> (unsigned 8bit integer=w289:u8[][])
                }
                frame Disabled {
                }
              }
              n117 = Round Toward -Infinity(1:w124) -> (0:w123:dbl[][])
              n118 = disable-structure shown="Enabled" {
                disable-tunnel: w143 -> [w287 w288]
                disable-tunnel: u8 8 ("y") -> [w286 _]
                disable-tunnel: [w283 w288] -> w152
                frame Enabled {
                  n119 = Divide(x=w287, y=w286) -> (x/y=w285:dbl[][])
                  n120 = Round Toward -Infinity(1:w285) -> (0:w284:dbl[][])
                  n121 = To Unsigned Byte Integer(number=w284) -> (unsigned 8bit integer=w283:u8[][])
                }
                frame Disabled {
                }
              }
              n122 = Round Toward -Infinity(1:w226) -> (0:w227:dbl[][])
              n123 = Divide(x=w131, y=w118) -> (x/y=w122:dbl[][])
              n124 = To Unsigned Byte Integer(number=w123) -> (unsigned 8bit integer=w133:u8[][])
              n125 = Round Toward -Infinity(1:w122) -> (0:w121:dbl[][])
              n126 = To Unsigned Byte Integer(number=w227) -> (unsigned 8bit integer=w219:u8[][])
              n127 = Increment(x=w133) -> (x+1=w128:u8[][])
              n128 = To Long Integer(number=w107) -> (32bit integer=w129:i32[][])
              n129 = Initialize Array(0.0 ("element"), 6 ("dimension size")) -> (w223:dbl[])
              n130 = To Unsigned Byte Integer(number=w121) -> (unsigned 8bit integer=w132:u8[][])
              n131 = call "IMAQ GetImageSize"("Image"=w181) -> ("Y Resolution"=w188:i32, "X Resolution"=w187:i32)  [unwired: 1 in, 3 out]
              n132 = Add Array Elements(numeric array=w129) -> (sum=w130:i32)
              n133 = call "IMAQ GetImageSize"("Image"=w162) -> ("Y Resolution"=w169:i32, "X Resolution"=w168:i32)  [unwired: 1 in, 3 out]
              n134 = Increment(x=w132) -> (x+1=w125:u8[][])
              n135 = Initialize Array(0.0 ("element"), 6 ("dimension size")) -> (w184:dbl[])
              n136 = dll-call lib="PTH2iabs E文章投稿&51. 代明球老师-玉米胁迫实验\tRGB程序maizeRealseHistProperty.dll" fn="HistProperty"(error in=w225, "Im"=w219, "row"=w230, "col"=w220, "G"=32, "HistStat"=w223) -> ("HistStat"=w63:dbl[])  [unwired: 6 in, 3 out]
              "HistStat_I" <- w63
              n137 = Initialize Array(0.0 ("element"), 6 ("dimension size")) -> (w165:dbl[])
              n138 = Initialize Array(sgl 0.0 ("element"), 15 ("dimension size")) -> (w136:sgl[])
              n139 = Initialize Array(sgl 0.0 ("element"), "level", "level") -> (w119:sgl[][])
              n140 = call "IMAQ GetImageSize"("Image"=w144) -> ("Y Resolution"=w151:i32, "X Resolution"=w150:i32)  [unwired: 1 in, 3 out]
              n141 = Initialize Array(0.0 ("element"), 6 ("dimension size")) -> (w147:dbl[])
              n142 = call "IMAQ Particle Analysis"("Pixel Measurements"=w101, "Image"=w77) -> ("Particle Measurements (Pixels)"=w81:dbl[][])  [unwired: 3 in, 6 out]
              n143 = call "IMAQ Particle Analysis"("Pixel Measurements"=w87, "Image"=w77) -> ("Particle Measurements (Pixels)"=w93:dbl[][])  [unwired: 3 in, 6 out]
              n144 = call "IMAQ Particle Analysis"("Pixel Measurements"=w92, "Image"=w77) -> ("Particle Measurements (Pixels)"=w98:dbl[][])  [unwired: 3 in, 6 out]
              n145 = call "IMAQ Particle Analysis"("Pixel Measurements"=w89, "Image"=w77) -> ("Particle Measurements (Pixels)"=w91:dbl[][])  [unwired: 3 in, 6 out]
              n146 = call "IMAQ Particle Analysis"("Pixel Measurements"=w85, "Image"=w77) -> ("Particle Measurements (Pixels)"=w83:dbl[][])  [unwired: 3 in, 6 out]
              n147 = dll-call lib="PTH2iabs E文章投稿&51. 代明球老师-玉米胁迫实验\tRGB程序maizeRealseHistProperty.dll" fn="HistProperty"(error in=w182, "Im"=w189, "row"=w188, "col"=w187, "G"=32, "HistStat"=w184) -> ("HistStat"=w62:dbl[])  [unwired: 6 in, 3 out]
              "HistStat_H" <- w62
              n148 = dll-call lib="PTH2iabs E文章投稿&51. 代明球老师-玉米胁迫实验\tRGB程序maizeRealseHistProperty.dll" fn="HistProperty"(error in=w163, "Im"=w170, "row"=w169, "col"=w168, "G"=32, "HistStat"=w165) -> ("HistStat"=w61:dbl[])  [unwired: 6 in, 3 out]
              "HistStat_G" <- w61
              n149 = dll-call lib="PTH2iabs E文章投稿&51. 代明球老师-玉米胁迫实验\tRGB程序maizeRealseHistProperty.dll" fn="HistProperty"(error in=w145, "Im"=w152, "row"=w151, "col"=w150, "G"=32, "HistStat"=w147) -> ("HistStat"=w60:dbl[])  [unwired: 6 in, 3 out]
              "HistStat_S" <- w60
              n150 = Add Array Elements(numeric array=w81) -> (sum=w80:dbl)
              n151 = Greater Or Equal?(x=w80, y=1000.0) -> (x >= y?=w78:bool)
              n152 = case shown="True" w78 {
                tunnel: [w236 w258] -> w57
                tunnel: [w236 w254] -> w55
                tunnel: [w236 w248] -> w54
                tunnel: [w236 w246] -> w53
                tunnel: [w236 w245] -> w56
                tunnel: w77 -> [_ w239]
                tunnel: [w236 w238] -> w58
                frame False {
                  w236 = 0.0 ("Numeric")
                }
                frame True {
                  w241 = T5[] [53] items=["Center of Mass X", "Center of Mass Y", "First Pixel X", "First Pixel Y", "Bounding Rect Left", "Bounding Rect Top", "Bounding Rect Right", "Bounding Rect Bottom", "Max Feret Diameter Start X", "Max Feret Diameter Start Y", "Max Feret Diameter End X", "Max Feret Diameter End Y", "Max Horiz. Segment Length Left", "Max Horiz. Segment Length Right", "Max Horiz. Segment Length Row", "-", "Bounding Rect Width", "Bounding Rect Height", "Bounding Rect Diagonal", "Perimeter", "Convex Hull Perimeter", "Holes' Perimeter", "Max Feret Diameter", "Equivalent Ellipse Major Axis", "Equivalent Ellipse Minor Axis", "Equivalent Ellipse Minor Axis (Feret)", "Equivalent Rect Long Side", "Equivalent Rect Short Side", "Equivalent Rect Diagonal", "Equivalent Rect Short Side (Feret)", "Average Horiz. Segment Length", "Average Vert. Segment Length", "Hydraulic Radius", "Waddel Disk Diameter", "-", "Area", "Holes' Area", "Particle & Holes' Area", "Convex Hull Area", "Image Area", "-", "Number of Holes", "Number of Horiz. Segments", "Number of Vert. Segments", "-", "Orientation", "Max Feret Diameter Orientation", "-", "% Area/Image Area", "% Area/(Particle & Holes' Area)", "Ratio of Equivalent Ellipse Axes", "Ratio of Equivalent Rect Sides", "-", "Elongation Factor", "Compactness Factor", "Heywood Circularity Factor", "Type Factor", "-", "Sum X", "Sum Y", "Sum XX", "Sum XY", "Sum YY", "Sum XXX", "Sum XXY", "Sum XYY", "Sum YYY", "-", "Moment of Inertia XX", "Moment of Inertia XY", "Moment of Inertia YY", "Moment of Inertia XXX", "Moment of Inertia XXY", "Moment of Inertia XYY", "Moment of Inertia YYY", "Norm. Moment of Inertia XX", "Norm. Moment of Inertia XY", "Norm. Moment of Inertia YY", "Norm. Moment of Inertia XXX", "Norm. Moment of Inertia XXY", "Norm. Moment of Inertia XYY", "Norm. Moment of Inertia YYY", "Hu Moment 1", "Hu Moment 2", "Hu Moment 3", "Hu Moment 4", "Hu Moment 5", "Hu Moment 6", "Hu Moment 7"] ("Pixel Measurements")
                  w263 = T5[] [56] items=["Center of Mass X", "Center of Mass Y", "First Pixel X", "First Pixel Y", "Bounding Rect Left", "Bounding Rect Top", "Bounding Rect Right", "Bounding Rect Bottom", "Max Feret Diameter Start X", "Max Feret Diameter Start Y", "Max Feret Diameter End X", "Max Feret Diameter End Y", "Max Horiz. Segment Length Left", "Max Horiz. Segment Length Right", "Max Horiz. Segment Length Row", "-", "Bounding Rect Width", "Bounding Rect Height", "Bounding Rect Diagonal", "Perimeter", "Convex Hull Perimeter", "Holes' Perimeter", "Max Feret Diameter", "Equivalent Ellipse Major Axis", "Equivalent Ellipse Minor Axis", "Equivalent Ellipse Minor Axis (Feret)", "Equivalent Rect Long Side", "Equivalent Rect Short Side", "Equivalent Rect Diagonal", "Equivalent Rect Short Side (Feret)", "Average Horiz. Segment Length", "Average Vert. Segment Length", "Hydraulic Radius", "Waddel Disk Diameter", "-", "Area", "Holes' Area", "Particle & Holes' Area", "Convex Hull Area", "Image Area", "-", "Number of Holes", "Number of Horiz. Segments", "Number of Vert. Segments", "-", "Orientation", "Max Feret Diameter Orientation", "-", "% Area/Image Area", "% Area/(Particle & Holes' Area)", "Ratio of Equivalent Ellipse Axes", "Ratio of Equivalent Rect Sides", "-", "Elongation Factor", "Compactness Factor", "Heywood Circularity Factor", "Type Factor", "-", "Sum X", "Sum Y", "Sum XX", "Sum XY", "Sum YY", "Sum XXX", "Sum XXY", "Sum XYY", "Sum YYY", "-", "Moment of Inertia XX", "Moment of Inertia XY", "Moment of Inertia YY", "Moment of Inertia XXX", "Moment of Inertia XXY", "Moment of Inertia XYY", "Moment of Inertia YYY", "Norm. Moment of Inertia XX", "Norm. Moment of Inertia XY", "Norm. Moment of Inertia YY", "Norm. Moment of Inertia XXX", "Norm. Moment of Inertia XXY", "Norm. Moment of Inertia XYY", "Norm. Moment of Inertia YYY", "Hu Moment 1", "Hu Moment 2", "Hu Moment 3", "Hu Moment 4", "Hu Moment 5", "Hu Moment 6", "Hu Moment 7"] ("Pixel Measurements")
                  w264 = T5[] [55] items=["Center of Mass X", "Center of Mass Y", "First Pixel X", "First Pixel Y", "Bounding Rect Left", "Bounding Rect Top", "Bounding Rect Right", "Bounding Rect Bottom", "Max Feret Diameter Start X", "Max Feret Diameter Start Y", "Max Feret Diameter End X", "Max Feret Diameter End Y", "Max Horiz. Segment Length Left", "Max Horiz. Segment Length Right", "Max Horiz. Segment Length Row", "-", "Bounding Rect Width", "Bounding Rect Height", "Bounding Rect Diagonal", "Perimeter", "Convex Hull Perimeter", "Holes' Perimeter", "Max Feret Diameter", "Equivalent Ellipse Major Axis", "Equivalent Ellipse Minor Axis", "Equivalent Ellipse Minor Axis (Feret)", "Equivalent Rect Long Side", "Equivalent Rect Short Side", "Equivalent Rect Diagonal", "Equivalent Rect Short Side (Feret)", "Average Horiz. Segment Length", "Average Vert. Segment Length", "Hydraulic Radius", "Waddel Disk Diameter", "-", "Area", "Holes' Area", "Particle & Holes' Area", "Convex Hull Area", "Image Area", "-", "Number of Holes", "Number of Horiz. Segments", "Number of Vert. Segments", "-", "Orientation", "Max Feret Diameter Orientation", "-", "% Area/Image Area", "% Area/(Particle & Holes' Area)", "Ratio of Equivalent Ellipse Axes", "Ratio of Equivalent Rect Sides", "-", "Elongation Factor", "Compactness Factor", "Heywood Circularity Factor", "Type Factor", "-", "Sum X", "Sum Y", "Sum XX", "Sum XY", "Sum YY", "Sum XXX", "Sum XXY", "Sum XYY", "Sum YYY", "-", "Moment of Inertia XX", "Moment of Inertia XY", "Moment of Inertia YY", "Moment of Inertia XXX", "Moment of Inertia XXY", "Moment of Inertia XYY", "Moment of Inertia YYY", "Norm. Moment of Inertia XX", "Norm. Moment of Inertia XY", "Norm. Moment of Inertia YY", "Norm. Moment of Inertia XXX", "Norm. Moment of Inertia XXY", "Norm. Moment of Inertia XYY", "Norm. Moment of Inertia YYY", "Hu Moment 1", "Hu Moment 2", "Hu Moment 3", "Hu Moment 4", "Hu Moment 5", "Hu Moment 6", "Hu Moment 7"] ("Pixel Measurements")
                  w265 = T5[] [54] items=["Center of Mass X", "Center of Mass Y", "First Pixel X", "First Pixel Y", "Bounding Rect Left", "Bounding Rect Top", "Bounding Rect Right", "Bounding Rect Bottom", "Max Feret Diameter Start X", "Max Feret Diameter Start Y", "Max Feret Diameter End X", "Max Feret Diameter End Y", "Max Horiz. Segment Length Left", "Max Horiz. Segment Length Right", "Max Horiz. Segment Length Row", "-", "Bounding Rect Width", "Bounding Rect Height", "Bounding Rect Diagonal", "Perimeter", "Convex Hull Perimeter", "Holes' Perimeter", "Max Feret Diameter", "Equivalent Ellipse Major Axis", "Equivalent Ellipse Minor Axis", "Equivalent Ellipse Minor Axis (Feret)", "Equivalent Rect Long Side", "Equivalent Rect Short Side", "Equivalent Rect Diagonal", "Equivalent Rect Short Side (Feret)", "Average Horiz. Segment Length", "Average Vert. Segment Length", "Hydraulic Radius", "Waddel Disk Diameter", "-", "Area", "Holes' Area", "Particle & Holes' Area", "Convex Hull Area", "Image Area", "-", "Number of Holes", "Number of Horiz. Segments", "Number of Vert. Segments", "-", "Orientation", "Max Feret Diameter Orientation", "-", "% Area/Image Area", "% Area/(Particle & Holes' Area)", "Ratio of Equivalent Ellipse Axes", "Ratio of Equivalent Rect Sides", "-", "Elongation Factor", "Compactness Factor", "Heywood Circularity Factor", "Type Factor", "-", "Sum X", "Sum Y", "Sum XX", "Sum XY", "Sum YY", "Sum XXX", "Sum XXY", "Sum XYY", "Sum YYY", "-", "Moment of Inertia XX", "Moment of Inertia XY", "Moment of Inertia YY", "Moment of Inertia XXX", "Moment of Inertia XXY", "Moment of Inertia XYY", "Moment of Inertia YYY", "Norm. Moment of Inertia XX", "Norm. Moment of Inertia XY", "Norm. Moment of Inertia YY", "Norm. Moment of Inertia XXX", "Norm. Moment of Inertia XXY", "Norm. Moment of Inertia XYY", "Norm. Moment of Inertia YYY", "Hu Moment 1", "Hu Moment 2", "Hu Moment 3", "Hu Moment 4", "Hu Moment 5", "Hu Moment 6", "Hu Moment 7"] ("Pixel Measurements")
                  w240 = T5[] [19] items=["Center of Mass X", "Center of Mass Y", "First Pixel X", "First Pixel Y", "Bounding Rect Left", "Bounding Rect Top", "Bounding Rect Right", "Bounding Rect Bottom", "Max Feret Diameter Start X", "Max Feret Diameter Start Y", "Max Feret Diameter End X", "Max Feret Diameter End Y", "Max Horiz. Segment Length Left", "Max Horiz. Segment Length Right", "Max Horiz. Segment Length Row", "-", "Bounding Rect Width", "Bounding Rect Height", "Bounding Rect Diagonal", "Perimeter", "Convex Hull Perimeter", "Holes' Perimeter", "Max Feret Diameter", "Equivalent Ellipse Major Axis", "Equivalent Ellipse Minor Axis", "Equivalent Ellipse Minor Axis (Feret)", "Equivalent Rect Long Side", "Equivalent Rect Short Side", "Equivalent Rect Diagonal", "Equivalent Rect Short Side (Feret)", "Average Horiz. Segment Length", "Average Vert. Segment Length", "Hydraulic Radius", "Waddel Disk Diameter", "-", "Area", "Holes' Area", "Particle & Holes' Area", "Convex Hull Area", "Image Area", "-", "Number of Holes", "Number of Horiz. Segments", "Number of Vert. Segments", "-", "Orientation", "Max Feret Diameter Orientation", "-", "% Area/Image Area", "% Area/(Particle & Holes' Area)", "Ratio of Equivalent Ellipse Axes", "Ratio of Equivalent Rect Sides", "-", "Elongation Factor", "Compactness Factor", "Heywood Circularity Factor", "Type Factor", "-", "Sum X", "Sum Y", "Sum XX", "Sum XY", "Sum YY", "Sum XXX", "Sum XXY", "Sum XYY", "Sum YYY", "-", "Moment of Inertia XX", "Moment of Inertia XY", "Moment of Inertia YY", "Moment of Inertia XXX", "Moment of Inertia XXY", "Moment of Inertia XYY", "Moment of Inertia YYY", "Norm. Moment of Inertia XX", "Norm. Moment of Inertia XY", "Norm. Moment of Inertia YY", "Norm. Moment of Inertia XXX", "Norm. Moment of Inertia XXY", "Norm. Moment of Inertia XYY", "Norm. Moment of Inertia YYY", "Hu Moment 1", "Hu Moment 2", "Hu Moment 3", "Hu Moment 4", "Hu Moment 5", "Hu Moment 6", "Hu Moment 7"] ("Pixel Measurements")
                  w266 = T5[] [35] items=["Center of Mass X", "Center of Mass Y", "First Pixel X", "First Pixel Y", "Bounding Rect Left", "Bounding Rect Top", "Bounding Rect Right", "Bounding Rect Bottom", "Max Feret Diameter Start X", "Max Feret Diameter Start Y", "Max Feret Diameter End X", "Max Feret Diameter End Y", "Max Horiz. Segment Length Left", "Max Horiz. Segment Length Right", "Max Horiz. Segment Length Row", "-", "Bounding Rect Width", "Bounding Rect Height", "Bounding Rect Diagonal", "Perimeter", "Convex Hull Perimeter", "Holes' Perimeter", "Max Feret Diameter", "Equivalent Ellipse Major Axis", "Equivalent Ellipse Minor Axis", "Equivalent Ellipse Minor Axis (Feret)", "Equivalent Rect Long Side", "Equivalent Rect Short Side", "Equivalent Rect Diagonal", "Equivalent Rect Short Side (Feret)", "Average Horiz. Segment Length", "Average Vert. Segment Length", "Hydraulic Radius", "Waddel Disk Diameter", "-", "Area", "Holes' Area", "Particle & Holes' Area", "Convex Hull Area", "Image Area", "-", "Number of Holes", "Number of Horiz. Segments", "Number of Vert. Segments", "-", "Orientation", "Max Feret Diameter Orientation", "-", "% Area/Image Area", "% Area/(Particle & Holes' Area)", "Ratio of Equivalent Ellipse Axes", "Ratio of Equivalent Rect Sides", "-", "Elongation Factor", "Compactness Factor", "Heywood Circularity Factor", "Type Factor", "-", "Sum X", "Sum Y", "Sum XX", "Sum XY", "Sum YY", "Sum XXX", "Sum XXY", "Sum XYY", "Sum YYY", "-", "Moment of Inertia XX", "Moment of Inertia XY", "Moment of Inertia YY", "Moment of Inertia XXX", "Moment of Inertia XXY", "Moment of Inertia XYY", "Moment of Inertia YYY", "Norm. Moment of Inertia XX", "Norm. Moment of Inertia XY", "Norm. Moment of Inertia YY", "Norm. Moment of Inertia XXX", "Norm. Moment of Inertia XXY", "Norm. Moment of Inertia XYY", "Norm. Moment of Inertia YYY", "Hu Moment 1", "Hu Moment 2", "Hu Moment 3", "Hu Moment 4", "Hu Moment 5", "Hu Moment 6", "Hu Moment 7"] ("Pixel Measurements")
                  w280 = T4 0 items=["Grayscale (U8)", "Grayscale (I16)", "Grayscale (SGL)", "Complex (CSG)", "RGB (U32)", "HSL (U32)", "RGB (U64)", "Grayscale (U16)"] ("Image Type")
                  n153 = call "IMAQ ImageToArray"("Image"=w239) -> ("Image Pixels (U8)"=w282:u8[][])  [unwired: 2 in, 5 out]
                  n154 = call "IMAQ GetImageSize"("Image"=w239) -> ("Y Resolution"=w273:i32, "X Resolution"=w272:i32)  [unwired: 1 in, 3 out]
                  n155 = Initialize Array(u8 0 ("element"), w273, w272) -> (w278:u8[][])
                  n156 = Initialize Array(u32 0 ("element"), w273, w272) -> (w274:u32[][])
                  n157 = dll-call lib="PTH2pabs E文章投稿&51. 代明球老师-玉米胁迫实验\tRGB程序maizeTotalContoursConvexHull (5).dll" fn="TotalContoursConvexHull"("src"=w282, "width"=w272, "height"=w273, "bwhullimage"=w278, "rgbhullimage"=w274) -> ("bwhullimage"=w276:u8[][])  [unwired: 7 in, 3 out]
                  n158 = call "IMAQ Create"("Image Name"="bwhullimage", "Image Type"=w280) -> ("New Image"=w279:T1)  [unwired: 2 in, 2 out]
                  n159 = call "IMAQ ArrayToImage"("Image Pixels (U8)"=w276, "Image"=w279) -> ("Image Out"=w267:T1)  [unwired: 4 in, 5 out]
                  n160 = call "IMAQ Threshold"("Range"=cluster{"Lower value":sgl, "Upper value":sgl} {"Lower value"=128.0, "Upper value"=255.0}, "Image Src"=w267) -> ("error out"=w270:errorcluster, "Image Dst Out"=w268:T1)  [unwired: 4 in, 4 out]
                  n161 = call "IMAQ FillHole"("error in (no error)"=w270, "Image Src"=w268, "Connectivity 4/8 (8)"=TRUE) -> ("Image Dst Out"=w237:T1)  [unwired: 1 in, 3 out]
                  "Convex Hull image" <- w237
                  n162 = call "IMAQ Particle Analysis"("Pixel Measurements"=w264, "Image"=w237) -> ("Particle Measurements (Pixels)"=w252:dbl[][], "Number of Particles"=w249:i32)  [unwired: 3 in, 5 out]
                  n163 = call "IMAQ Particle Analysis"("Pixel Measurements"=w263, "Image"=w237) -> ("Particle Measurements (Pixels)"=w250:dbl[][], "Number of Particles"=w247:i32)  [unwired: 3 in, 5 out]
                  n164 = call "IMAQ Particle Analysis"("Pixel Measurements"=w241, "Image"=w237) -> ("Particle Measurements (Pixels)"=w243:dbl[][], "Number of Particles"=w244:i32)  [unwired: 3 in, 5 out]
                  n165 = call "IMAQ Particle Analysis"("Pixel Measurements"=w266, "Image"=w237) -> ("Particle Measurements (Pixels)"=w262:dbl[][])  [unwired: 3 in, 6 out]
                  n166 = call "IMAQ Particle Analysis"("Pixel Measurements"=w265, "Image"=w237) -> ("Particle Measurements (Pixels)"=w256:dbl[][], "Number of Particles"=w255:i32)  [unwired: 3 in, 5 out]
                  n167 = call "IMAQ Particle Analysis"("Pixel Measurements"=w240, "Image"=w237) -> ("Particle Measurements (Pixels)"=w261:dbl[][], "Number of Particles"=w259:i32)  [unwired: 3 in, 5 out]
                  n168 = Add Array Elements(numeric array=w250) -> (sum=w251:dbl)
                  n169 = Add Array Elements(numeric array=w243) -> (sum=w242:dbl)
                  n170 = Add Array Elements(numeric array=w252) -> (sum=w253:dbl)
                  n171 = Add Array Elements(numeric array=w261) -> (sum=w260:dbl)
                  n172 = Add Array Elements(numeric array=w256) -> (sum=w257:dbl)
                  n173 = Divide(x=w251, y=w247) -> (x/y=w246:dbl)
                  n174 = Divide(x=w242, y=w244) -> (x/y=w245:dbl)
                  n175 = Add Array Elements(numeric array=w262) -> (sum=w238:dbl)
                  n176 = Divide(x=w253, y=w249) -> (x/y=w248:dbl)
                  n177 = Divide(x=w260, y=w259) -> (x/y=w258:dbl)
                  n178 = Divide(x=w257, y=w255) -> (x/y=w254:dbl)
                }
              }
              "Area_convex hull" <- w58
              "Perimeter_convex hull" <- w57
              "Elongation_convex hull" <- w56
              "Compactness_convex hull" <- w55
              "Heywood_convex hull" <- w54
              "Type_convex hull" <- w53
              n179 = Index Array(array=w81, index (col)=0 ("disabled index (col)")) -> (element=w99:dbl[])  [unwired: 1 in]
              n180 = Index Array(array=w93, index (col)=0 ("disabled index (col)")) -> (element=w95:dbl[])  [unwired: 1 in]
              n181 = Index Array(array=w98, index (col)=0 ("disabled index (col)")) -> (element=w96:dbl[])  [unwired: 1 in]
              n182 = Index Array(array=w91, index (col)=0 ("disabled index (col)")) -> (element=w88:dbl[])  [unwired: 1 in]
              n183 = Index Array(array=w83, index (col)=0 ("disabled index (col)")) -> (element=w86:dbl[])  [unwired: 1 in]
              n184 = dll-call lib="PTH2Yabs E文章投稿&51. 代明球老师-玉米胁迫实验\tRGB程序maizeGLCM.dll" fn="createGLCM"("G"=w128, "Grad"=w125, "mask"=w107, "row"=w109, "col"=w108, "level"=w126, "N"=w130, "T"=w136, "glcm"=w119) -> ("T"=w59:sgl[])  [unwired: 11 in, 3 out]
              "T" <- w59
              n185 = Array Max & Min(array=w99) -> (max index (indices)=w82:i32)  [unwired: 3 out]
              n186 = Index Array(array=w95, index=w82) -> (element=w51:dbl)
              "Compactness" <- w51
              n187 = Index Array(array=w96, index=w82) -> (element=w52:dbl)
              "Elongation" <- w52
              n188 = Index Array(array=w88, index=w82) -> (element=w50:dbl)
              "Heywood" <- w50
              n189 = Index Array(array=w86, index=w82) -> (element=w49:dbl)
              "Type" <- w49
              n190 = Divide(x=w203, y=w201) -> (x/y=w65:dbl)
              "GCV2" <- w65
              n191 = Divide(x=w80, y=w58) -> (x/y=w48:dbl)
              "Area/convex hull area" <- w48
              n192 = Build Array (concatenate)(w45, w75, w74, w73, w72, w71, w70, w69, w68, w67, w66, w65) -> (w64:dbl[])
              n193 = Build Array(w58, w57, w56, w55, w54, w53, w52, w51, w50, w49, w48) -> (w47:dbl[])
              n194 = Build Array (concatenate)(w64, w63, w62, w61, w60, w59, w47) -> (w46:dbl[])
            }
          }
        }
        frame #1 {
          n195 = case shown="True" w325 {
            tunnel: w337 -> [_ w340]
            tunnel: w327 -> [_ w364]
            tunnel: [dbl[] [] w360] -> w326
            tunnel: w324 -> [_ w355]
            frame False {
            }
            frame True {
              w349 = T4 0 items=["Grayscale (U8)", "Grayscale (I16)", "Grayscale (SGL)", "Complex (CSG)", "RGB (U32)", "HSL (U32)", "RGB (U64)", "Grayscale (U16)"] ("Image Type")
              # "去除小区域"
              n196 = call "IMAQ FillHole"("Image Src"=w340) -> ("Image Dst Out"=w339:T1)  [unwired: 3 in, 3 out]
              n197 = call "IMAQ GetImageSize"("Image"=w339) -> ("Y Resolution"=w345:i32, "X Resolution"=w344:i32)  [unwired: 1 in, 3 out]
              n198 = call "IMAQ ImageToArray"("Image"=w339) -> ("Image Pixels (U8)"=w343:u8[][])  [unwired: 2 in, 5 out]
              n199 = Initialize Array(0.0 ("element"), 40 ("dimension size")) -> (w461:dbl[])
              n200 = Initialize Array(0.0 ("element"), 40 ("dimension size")) -> (w458:dbl[])
              n201 = Initialize Array(u32 0 ("element"), 40 ("dimension size")) -> (w418:u32[])
              n202 = Initialize Array(i8 0 ("element"), 40 ("dimension size")) -> (w464:i8[])
              n203 = Initialize Array(0.0 ("element"), 40 ("dimension size")) -> (w414:dbl[])
              n204 = Initialize Array(0.0 ("element"), 40 ("dimension size")) -> (w453:dbl[])
              n205 = call "IMAQ Create"("Image Name"="remove_final", "Image Type"=w349) -> ("New Image"=w347:T1)  [unwired: 2 in, 2 out]
              n206 = dll-call lib="PTH2iabs E文章投稿&51. 代明球老师-玉米胁迫实验\tRGB程序maizeRealseimFillRemove.dll" fn="bwremove"("bw"=w343, "row"=w345, "col"=w344, "areathreshold"=1000) -> ("bw"=w346:u8[][])  [unwired: 6 in, 3 out]
              n207 = call "IMAQ ArrayToImage"("Image Pixels (U8)"=w346, "Image"=w347) -> ("Image Out"=w341:T1)  [unwired: 4 in, 5 out]
              n208 = call "IMAQ Morphology"("Number of iterations (1)"=1, "Square/Hexa (Square)"=FALSE, "Operation"=T2."Dilate", "Image Src"=w341) -> ("Image Dst Out"=w350:T1)  [unwired: 3 in, 4 out]
              n209 = call "IMAQ GetImageSize"("Image"=w341) -> ("Y Resolution"=w403:i32, "X Resolution"=w402:i32)  [unwired: 1 in, 3 out]
              n210 = Initialize Array(u8 0 ("element"), w403, w402) -> (w451:u8[][])
              n211 = call "IMAQ ImageToArray"("Image"=w350) -> ("Image Pixels (U8)"=w468:u8[][])  [unwired: 2 in, 5 out]
              n212 = disable-structure shown="Enabled" {
                disable-tunnel: w468 -> [w515 _]
                disable-tunnel: u32 0 ("outputLeafNum") -> [w514 _]
                disable-tunnel: w464 -> [w513 _]
                disable-tunnel: w461 -> [w512 _]
                disable-tunnel: w458 -> [w511 _]
                disable-tunnel: w453 -> [w510 _]
                disable-tunnel: w451 -> [w508 _]
                disable-tunnel: [w507 _] -> w450
                disable-tunnel: [w506 _] -> w449
                disable-tunnel: [w505 _] -> w448
                disable-tunnel: [w504 _] -> w447
                disable-tunnel: [w503 _] -> w423
                disable-tunnel: [w502 _] -> w421
                disable-tunnel: [w501 _] -> w419
                disable-tunnel: w418 -> [w500 _]
                disable-tunnel: [w499 _] -> w417
                disable-tunnel: w414 -> [w498 _]
                disable-tunnel: 0.0 ("steamWidth") -> [w497 _]
                disable-tunnel: [w496 _] -> w412
                disable-tunnel: w403 -> [w495 _]
                disable-tunnel: w402 -> [w494 _]
                disable-tunnel: [w493 _] -> w389
                disable-tunnel: [w492 _] -> w385
                frame Disabled {
                  n213 = dll-call lib="E:/maize/FTKToolkit_CPP_VC8.dll" fn="maizeSingleLeafExtraction_auto"("inputImageData"=w515, "inputImageRw"=w495, "inputImageCol"=w494, "outputLeafNum"=w514, "inputLeafEndPoint"=w513, "leafAngle1"=w512, "leafAngle2"=w511, "nodePointPosition"=w500, "leafLength"=w510, "leafEndToEndDistance"=w498, "steamWidth"=w497, "matPlane2"=w508, "matPlane1"=w508, "matPlane0"=w508, "debug"=u8 0) -> ("outputLeafNum"=w493:u32, "inputLeafEndPoint"=w504:u32[], "leafAngle1"=w503:dbl[], "leafAngle2"=w502:dbl[], "nodePointPosition"=w499:u32[], "leafLength"=w501:dbl[], "leafEndToEndDistance"=w496:dbl[], "steamWidth"=w492:dbl, "matPlane2"=w507:u8[][], "matPlane1"=w506:u8[][], "matPlane0"=w505:u8[][])  [unwired: 7 in, 3 out]
                }
                frame Enabled {
                }
              }
              "outputLeafNum" <- w389
              "inputLeafEndPoint" <- w447
              "leafAngle1" <- w423
              "leafAngle2" <- w421
              "nodePointPosition" <- w417
              "leafLength" <- w419
              "leafEndToEndDistance" <- w412
              "steamWidth" <- w385
              n214 = Search/Split String(string=w355, search string/char (-)=".png") -> (substring before match=w358:string, match + rest of string=w356:string)  [unwired: 2 out]
              n215 = Concatenate Strings(w358, "_SK" ("string"), w356) -> (w354:string)
              n216 = disable-structure shown="Disabled" {
                disable-tunnel: w450 -> [w488 _]
                disable-tunnel: w449 -> [w481 _]
                disable-tunnel: w448 -> [w480 _]
                disable-tunnel: w354 -> [w470 _]
                frame Disabled {
                  w473 = u16 0 items=["RGB", "HSL", "HSV", "HSI"] ("Color Mode")
                  w479 = T4 4 items=["Grayscale (U8)", "Grayscale (I16)", "Grayscale (SGL)", "Complex (CSG)", "RGB (U32)", "HSL (U32)", "RGB (U64)", "Grayscale (U16)"] ("Image Type")
                  w483 = T4 0 items=["Grayscale (U8)", "Grayscale (I16)", "Grayscale (SGL)", "Complex (CSG)", "RGB (U32)", "HSL (U32)", "RGB (U64)", "Grayscale (U16)"] ("Image Type")
                  w486 = T4 0 items=["Grayscale (U8)", "Grayscale (I16)", "Grayscale (SGL)", "Complex (CSG)", "RGB (U32)", "HSL (U32)", "RGB (U64)", "Grayscale (U16)"] ("Image Type")
                  w490 = T4 0 items=["Grayscale (U8)", "Grayscale (I16)", "Grayscale (SGL)", "Complex (CSG)", "RGB (U32)", "HSL (U32)", "RGB (U64)", "Grayscale (U16)"] ("Image Type")
                  n217 = call "IMAQ Create"("Image Name"="skeleton_R", "Image Type"=w490) -> ("New Image"=w489:T1)  [unwired: 2 in, 2 out]
                  n218 = call "IMAQ Create"("Image Name"="skeleton_B", "Image Type"=w483) -> ("New Image"=w482:T1)  [unwired: 2 in, 2 out]
                  n219 = call "IMAQ Create"("Image Name"="skeleton_G", "Image Type"=w486) -> ("New Image"=w487:T1)  [unwired: 2 in, 2 out]
                  n220 = local read "Path of segmented images storage"() -> (w471:path)
                  n221 = call "IMAQ ArrayToImage"("Image Pixels (U8)"=w488, "Image"=w489) -> ("Image Out"=w475:T1)  [unwired: 4 in, 5 out]
                  n222 = call "IMAQ ArrayToImage"("Image Pixels (U8)"=w480, "Image"=w482) -> ("Image Out"=w474:T1)  [unwired: 4 in, 5 out]
                  n223 = call "IMAQ ArrayToImage"("Image Pixels (U8)"=w481, "Image"=w487) -> ("Image Out"=w476:T1)  [unwired: 4 in, 5 out]
                  n224 = call "IMAQ Create"("Image Name"="skeleton_RGB", "Image Type"=w479) -> ("New Image"=w477:T1)  [unwired: 2 in, 2 out]
                  n225 = call "IMAQ ReplaceColorPlane"("Color Mode"=w473, "Image Dst"=w477, "Red or Hue Plane"=w475, "Green or Sat Plane"=w474, "Blue or Luma or Val or Inten Plane"=w476) -> ("Image Dst Out"=w472:T1)  [unwired: 2 in, 8 out]
                  n226 = Build Path(base path=w471, name or relative path=w470) -> (appended path=w469:path)
                  n227 = call-poly "IMAQ Write File 2"("File Path"=w469, "Image"=w472) -> ()  [unwired: 4 in, 6 out]
                }
                frame Enabled {
                }
              }
              n228 = Array Subset(array=w421, length=w389) -> (w420:dbl[])  [unwired: 1 in]
              n229 = Array Subset(array=w423, length=w389) -> (w422:dbl[])  [unwired: 1 in]
              n230 = Array Subset(array=w419, length=w389) -> (w411:dbl[])  [unwired: 1 in]
              n231 = Array Subset(array=w412, length=w389) -> (w408:dbl[])  [unwired: 1 in]
              n232 = Multiply(x=w389, y=u32 2) -> (x*y=w445:u32)
              n233 = Divide(x=w408, y=w411) -> (x/y=w404:dbl[])
              n234 = Array Subset(array=w417, length=w445) -> (w444:u32[])  [unwired: 1 in]
              n235 = Quotient & Remainder(x=w389, y=2.0) -> (x-y*floor(x/y)=w433:dbl)  [unwired: 1 out]
              n236 = Not Equal?(x=w433, y=0.0) -> (x != y?=w431:bool)
              n237 = case shown="True" w431 {
                tunnel: w389 -> [w517 w523]
                tunnel: [w516 w519] -> w430
                frame False {
                  n238 = Divide(x=w517, y=2.0) -> (x/y=w516:dbl)
                }
                frame True {
                  n239 = Add(x=w523, y=1.0) -> (x+y=w521:dbl)
                  n240 = Divide(x=w521, y=2.0) -> (x/y=w519:dbl)
                }
              }
              n241 = call <vilib>:"Std Deviation and Variance.vi"("X"=w422) -> ("mean"=w401:dbl, "standard deviation"=w400:dbl)  [unwired: 1 in, 1 out]
              "叶片角度1总长(切线)" <- w401
              "叶片角度1标准差(切线)" <- w400
              n242 = call <vilib>:"Std Deviation and Variance.vi"("X"=w420) -> ("mean"=w399:dbl, "standard deviation"=w398:dbl)  [unwired: 1 in, 1 out]
              "叶片角度2总长" <- w399
              "叶片角度2标准差" <- w398
              n243 = Add Array Elements(numeric array=w411) -> (sum=w397:dbl)
              "拉直后叶长总长" <- w397
              n244 = Add Array Elements(numeric array=w408) -> (sum=w394:dbl)
              "叶尖点到结点总长" <- w394
              n245 = call <vilib>:"Std Deviation and Variance.vi"("X"=w411) -> ("mean"=w396:dbl, "standard deviation"=w395:dbl)  [unwired: 1 in, 1 out]
              "拉直后叶长均值" <- w396
              "拉直后叶长标准差" <- w395
              n246 = call <vilib>:"Std Deviation and Variance.vi"("X"=w408) -> ("mean"=w393:dbl, "standard deviation"=w392:dbl)  [unwired: 1 in, 1 out]
              "叶尖点到结点长度均值" <- w393
              "叶尖点到结点长度标准差" <- w392
              n247 = call <vilib>:"Std Deviation and Variance.vi"("X"=w404) -> ("mean"=w391:dbl, "standard deviation"=w390:dbl)  [unwired: 1 in, 1 out]
              "LC均值" <- w391
              "LC标准差" <- w390
              n248 = for {
                N: w389 -> [_]
                tunnel: w444 -> [w559]
                tunnel: [w557] -> w441 mode=indexing
                i -> [w561]
                n249 = Multiply(x=2, y=w561) -> (x*y=w558:i32)
                n250 = Index Array(array=w559, index=w558) -> (element=w557:u32)
              }
              n251 = for {
                N: w389 -> [_]
                tunnel: w444 -> [w554]
                tunnel: [w553] -> w443 mode=indexing
                i -> [w556]
                n252 = Multiply(x=2, y=w556) -> (x*y=w552:i32)
                n253 = Add(x=1, y=w552) -> (x+y=w550:i32)
                n254 = Index Array(array=w554, index=w550) -> (element=w553:u32)
              }
              n255 = To Unsigned Byte Integer(number=w430) -> (unsigned 8bit integer=w405:u8)
              "unsigned 8bit integer" <- w405
              n256 = Delete From Array(array=w420, length=w405) -> (deleted portion=w427:dbl[], array with subset deleted=w426:dbl[])  [unwired: 1 in]
              n257 = Delete From Array(array=w422, length=w405) -> (deleted portion=w428:dbl[], array with subset deleted=w429:dbl[])  [unwired: 1 in]
              "array w/ subset deleted" <- w429
              "deleted portion" <- w428
              n258 = Delete From Array(array=w411, length=w405) -> (deleted portion=w424:dbl[], array with subset deleted=w425:dbl[])  [unwired: 1 in]
              n259 = Delete From Array(array=w404, length=w405) -> (deleted portion=w406:dbl[], array with subset deleted=w407:dbl[])  [unwired: 1 in]
              n260 = Delete From Array(array=w408, length=w405) -> (deleted portion=w410:dbl[], array with subset deleted=w409:dbl[])  [unwired: 1 in]
              n261 = call <vilib>:"Std Deviation and Variance.vi"("X"=w426) -> ("mean"=w380:dbl, "standard deviation"=w379:dbl)  [unwired: 1 in, 1 out]
              "叶片角度2上半部分均值" <- w380
              "叶片角度2上半部分标准差" <- w379
              n262 = call <vilib>:"Std Deviation and Variance.vi"("X"=w429) -> ("mean"=w384:dbl, "standard deviation"=w383:dbl)  [unwired: 1 in, 1 out]
              "叶片角度1上半部分均值" <- w384
              "叶片角度1上半部分标准差" <- w383
              n263 = call <vilib>:"Std Deviation and Variance.vi"("X"=w427) -> ("mean"=w378:dbl, "standard deviation"=w377:dbl)  [unwired: 1 in, 1 out]
              "叶片角度2下半部分均值" <- w378
              "叶片角度2下半部分标准差" <- w377
              n264 = call <vilib>:"Std Deviation and Variance.vi"("X"=w428) -> ("mean"=w382:dbl, "standard deviation"=w381:dbl)  [unwired: 1 in, 1 out]
              "叶片角度1下半部分均值" <- w382
              "叶片角度1下半部分标准差" <- w381
              n265 = call <vilib>:"Std Deviation and Variance.vi"("X"=w425) -> ("mean"=w376:dbl, "standard deviation"=w375:dbl)  [unwired: 1 in, 1 out]
              "拉直后叶长上半部分均值" <- w376
              "拉直后叶长上半部分标准差" <- w375
              n266 = call <vilib>:"Std Deviation and Variance.vi"("X"=w407) -> ("mean"=w368:dbl, "standard deviation"=w367:dbl)  [unwired: 1 in, 1 out]
              "LC上半部分均值" <- w368
              "LC上半部分标准差" <- w367
              n267 = call <vilib>:"Std Deviation and Variance.vi"("X"=w409) -> ("mean"=w372:dbl, "standard deviation"=w371:dbl)  [unwired: 1 in, 1 out]
              "叶尖点到结点长度上半部分均值" <- w372
              "叶尖点到结点长度上半部分标准差" <- w371
              n268 = call <vilib>:"Std Deviation and Variance.vi"("X"=w424) -> ("mean"=w374:dbl, "standard deviation"=w373:dbl)  [unwired: 1 in, 1 out]
              "拉直后叶长下半部分均值" <- w374
              "拉直后叶长下半部分标准差" <- w373
              n269 = call <vilib>:"Std Deviation and Variance.vi"("X"=w406) -> ("mean"=w366:dbl, "standard deviation"=w365:dbl)  [unwired: 1 in, 1 out]
              "LC下半部分均值" <- w366
              "LC下半部分标准差" <- w365
              n270 = call <vilib>:"Std Deviation and Variance.vi"("X"=w410) -> ("mean"=w370:dbl, "standard deviation"=w369:dbl)  [unwired: 1 in, 1 out]
              "叶尖点到结点长度下半部分均值" <- w370
              "叶尖点到结点长度下半部分标准差" <- w369
              n271 = for {
                N: w389 -> [_]
                shift-right: [w545] -> _
                shift-left: w443 -> [w546]
                shift-right: [w548] -> w436
                shift-left: u32[] [] -> [w547]
                shift-right: [w540] -> w437
                shift-left: u32[] [] -> [w541]
                shift-right: [w542] -> _
                shift-left: w441 -> [w543]
                # "冒泡排序"
                n272 = Array Max & Min(array=w546) -> (max value=w549:u32, max index (indices)=w539:i32)  [unwired: 2 out]
                n273 = Index Array(array=w543, index=w539) -> (element=w544:u32)
                n274 = Delete From Array(array=w546, index=w539) -> (array with subset deleted=w545:u32[])  [unwired: 1 in, 1 out]
                n275 = Insert Into Array(array=w547, new element=w549) -> (w548:u32[])  [unwired: 1 in]
                n276 = Insert Into Array(array=w541, new element=w544) -> (w540:u32[])  [unwired: 1 in]
                n277 = Delete From Array(array=w543, index=w539) -> (array with subset deleted=w542:u32[])  [unwired: 1 in, 1 out]
              }
              n278 = Build Array(w401, w400, w399, w398, w397, w396, w395, w394, w393, w392, w391, w390) -> (w362:dbl[])
              n279 = Build Array(w384, w383, w382, w381, w380, w379, w378, w377, w376, w375, w374, w373, w372, w371, w370, w369, w368, w367, w366, w365) -> (w361:dbl[])
              n280 = Subtract(x=w389, y=u32 1) -> (x-y=w438:u32)
              n281 = for {
                N: w438 -> [_]
                tunnel: w437 -> [w536]
                tunnel: w436 -> [w535]
                tunnel: [w524] -> w435 mode=indexing
                i -> [w534]
                n282 = Add(x=1, y=w534) -> (x+y=w537:i32)
                n283 = Index Array(array=w536, index=w534) -> (element=w533:u32)
                n284 = Index Array(array=w536, index=w537) -> (element=w532:u32)
                n285 = Index Array(array=w535, index=w534) -> (element=w529:u32)
                n286 = Index Array(array=w535, index=w537) -> (element=w528:u32)
                n287 = Subtract(x=w533, y=w532) -> (x-y=w531:u32)
                n288 = Subtract(x=w529, y=w528) -> (x-y=w530:u32)
                n289 = Square(x=w531) -> (x^2=w527:u32)
                n290 = Square(x=w530) -> (x^2=w526:u32)
                n291 = Add(x=w527, y=w526) -> (x+y=w525:u32)
                n292 = Square Root(x=w525) -> (sqrt(x)=w524:dbl)
              }
              n293 = Add Array Elements(numeric array=w435) -> (sum=w388:dbl)
              "结点总长" <- w388
              n294 = call <vilib>:"Std Deviation and Variance.vi"("X"=w435) -> ("mean"=w387:dbl, "standard deviation"=w386:dbl)  [unwired: 1 in, 1 out]
              "结点长均值" <- w387
              "结点长标准差" <- w386
              n295 = Build Array(w389, w388, w387, w386, w385) -> (w363:dbl[])
              n296 = Build Array (concatenate)(w364, w363, w362, w361) -> (w360:dbl[])
            }
          }
          n297 = local read "Date"() -> (w330:string)
          n298 = Concatenate Strings(w330, ".txt" ("string")) -> (w335:string)
          n299 = Number To Fractional String(number=w326) -> (F-format string=w328:string[])  [unwired: 3 out]
          n300 = Build Path(base path="Path of data sotrage", name or relative path=w335) -> (appended path=w334:path)
          n301 = Build Array (concatenate)(w329, w328) -> (w332:string[])
          n302 = call-poly <vilib>:"Write To Spreadsheet File.vi"("append to file? (new file:F)"=TRUE, "1D data"=w332, "file path (dialog if empty)"=w334) -> ()  [unwired: 3 in, 3 out]
        }
      }
    }
  }
